vi "Process.vi"(8 "error in":errorcluster, 11 "MeasurementSMO":refnum<class "AFM_Litho_Plugin.IV.lvclass">) -> (0 "error out":errorcluster, 3 "MeasurementSMO out":refnum<class "AFM_Litho_Plugin.IV.lvclass">)   [LabVIEW 2019, in "AFM_Litho_Plugin.IV.lvclass"]
doc: "---------------------------------------------------------------\nJKI State Machine Objects™\nhttp://jki.net/state-machine-objects/\nCopyright (C) 2005-2015, JKI <info@jki.net>\nALL RIGHTS RESERVED"
uses:
  AFM_Litho_Plugin.IV.lvclass
  C:/Program Files (x86)/National Instruments/LabVIEW 2019/vi.lib/JKI/JKI SMO/SMO/SMO.lvclass
  C:/Program Files (x86)/National Instruments/LabVIEW 2019/vi.lib/JKI/JKI SMO/SMO.UI/SMO.UI.lvclass
  <vilib>/JKI/JKI SMO/SMO/Typedefs/Parent Call--Enum.ctl
  AFM_Litho_Plugin.IV.lvclass/AFM_Litho_Plugin.IV.ctl
  Typedefs/PrivateEvents--AFM_Litho_Plugin.IV.IV Run--Local.ctl
  <userlib>/LevyLab/Instrument Framework/SMOs/RemoteControl/RemoteControl.lvclass
  <userlib>/LevyLab/Instrument Framework/SMOs/RemoteControl/Typedefs/Message--Cluster.ctl
  <userlib>/LevyLab/Instrument Framework/SMOs/RemoteControl/Typedefs/PrivateEvents--RemoteControl.SendMessageToProcess.ctl
  Program Files (x86)/National Instruments/LabVIEW 2020/user.lib/LevyLab/Lockin-Multichannel/Instrument.DAQ/Typedefs/Get State-enum.ctl
  <vilib>/JKI/JKI SMO/SMO/SMO.lvclass/SMO.ctl
  <userlib>/LevyLab/Instrument Framework/SMOs/RemoteControl/Typedefs/RC Com Type--enum.ctl
  fb8dc625-7147-424d-9f65-00a13242d459.vi
  <vilib>/JKI/JKI SMO/SMO/Private/ReftoDVR--SMO.vi
  fb8dc625-7147-424d-9f65-00a13242d459.vi/a9304a9f-69c7-45ea-b89b-09982a2100b8.vi
  <vilib>/Utility/LVClass/Get LV Class Name.vi
  <vilib>/JDP Science/JSONtext/JSON text to Variant.vi
  <vilib>/JDP Science/JSONtext/LVClass Serializer/JSONtext LVClass Serializer.lvclass
  <vilib>/JKI/JKI SMO/SMO.UI/SMO.UI.lvclass
  <vilib>/JKI/JKI SMO/SMO/SMO.lvclass
  <userlib>/LevyLab/Lockin-Multichannel/Instrument.DAQ/Instrument.DAQ.lvclass
panel:
  out "Lock-in Connection":bool
  out "Incoming Command":string
  out "Start":dbl caption="Numeric"
  out "End":dbl caption="Numeric"
  out "Rate":dbl caption="Numeric"
  out "Cycles":u32 caption="Numeric"
  out "Pattern":T1(ring) caption="Enum"
  in  "Output Channel":u16(ring) caption="Ring" items=["Ring", "Item 1", "Item 2", "Item 3"]
  out "IV Plug-in Address":u32 caption="Numeric"
  in  "Lock-in Amplifier Address":string
  # "IV Curve Measurement Plugin"
  # "ipconfig /all"
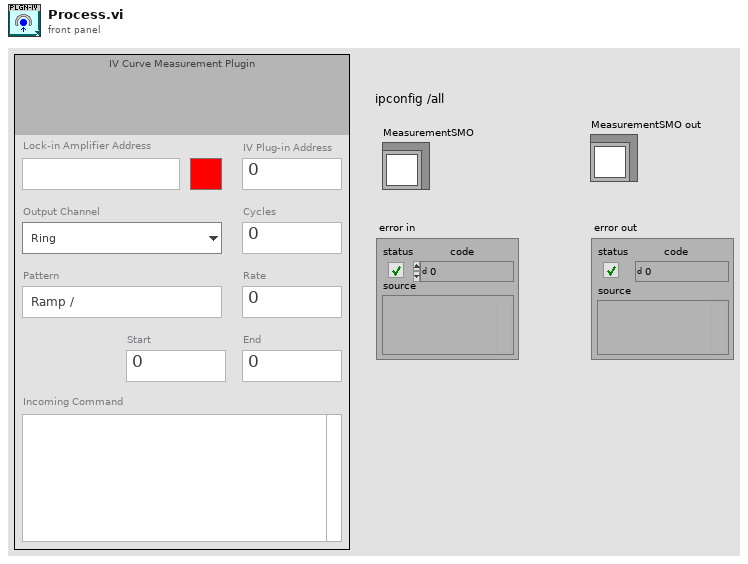
[diagram p1: front panel]
types:
  T1 = enum16{"Ramp /", "Ramp /\\", "Smooth Ramp _/", "Smooth Ramp _/\\_", "Frequency"}
  T2 = typedef "SMO.lvclass/Parent Call--Enum.ctl" = enum16{"Allows parent to run", "Does not request parent to run"}
  T3 = typedef "AFM_Litho_Plugin.IV.lvclass/PrivateEvents--AFM_Litho_Plugin.IV.IV Run--Local.ctl" = cluster{"Pattern":enum16{"Ramp /", "Ramp /\\", "Smooth Ramp _/", "Smooth Ramp _/\\_", "Frequency"}, "Cycles":dbl, "Rate":dbl, "End":dbl, "Start":dbl}
  T4 = enum32{"invalid app kind", "Development System", "Run Time System", "Student Edition", "Embedded LabVIEW", "Evaluation", "Custom"}
  T5 = typedef "Instrument.DAQ.lvclass/Get State-enum.ctl" = enum16{"idle", "created", "started", "stopped", "sweeping"}
  T6 = enum32{"Invalid", "Standard", "Closed", "Hidden", "Minimized", "Maximized"}
  T7 = enum32{"Bad", "Idle", "Run top level", "Running"}
  T8 = typedef "RemoteControl.lvclass/Message--Cluster.ctl" = cluster{"Command":string, "Data":variant, "ID":string}
  T9 = typedef "RemoteControl.lvclass/RC Com Type--enum.ctl" = enum16{"RC", "STM", "ZMQ"}
  T10 = cluster{"Shift":bool, "Ctrl":bool, "Alt":bool, "Cmd":bool, "Opt":bool}
  T11 = typedef "RemoteControl.lvclass/PrivateEvents--RemoteControl.SendMessageToProcess.ctl" = cluster{"Message":T8}
  T12 = cluster{"Core":cluster{"Current VI Reference":refnum<vi>, "Close Panel on Exit?":bool, "error":errorcluster}, "Self Reference":refnum<class "AFM_Litho_Plugin.IV.lvclass">, "Voltage Channel":u16, "Lockin Address":string, "Plugin Address":i32, "Server":refnum<class "RemoteControl.lvclass">, "Server Req":T8, "Server Rep":T11, "Cycles":dbl, "Status":T5, "IV Run":T3, "IV Status":string, "Command History":string, "Command Message":string, "Start Status":string}
  T13 = cluster{"Current VI Reference":refnum<vi>, "Close Panel on Exit?":bool, "error":errorcluster}
  T14 = typedef "RemoteControl.lvclass/PublicEvents--Cluster.ctl" = cluster{"SendMessageFromProcess":refnum<user-event>}
  T15 = typedef "AFM_Litho_Plugin.IV.lvclass/PrivateEvents--Cluster.ctl" = cluster{"IV Run--Local":refnum<user-event>, "IV Status--Local":refnum<user-event>}
  T16 = typedef "SMO.lvclass/Protected Events.ctl" = cluster{"StopProcesses":refnum<user-event>, "AbortProcesses":refnum<user-event>, "Config Changed":refnum<user-event>, "Dependency":refnum<user-event>}
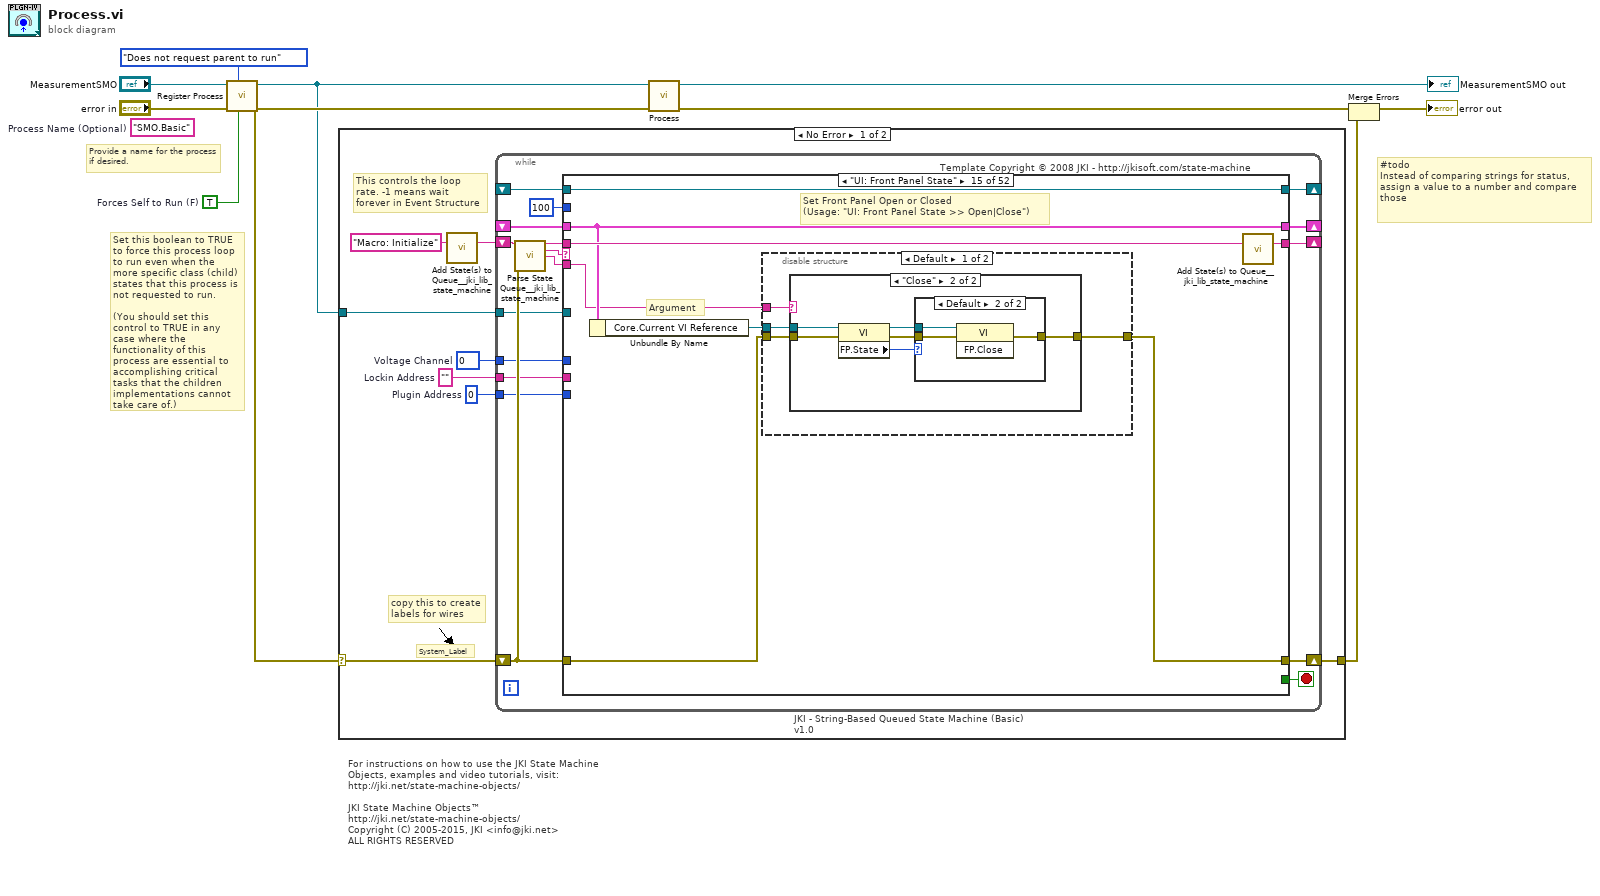
[diagram p0: block diagram]
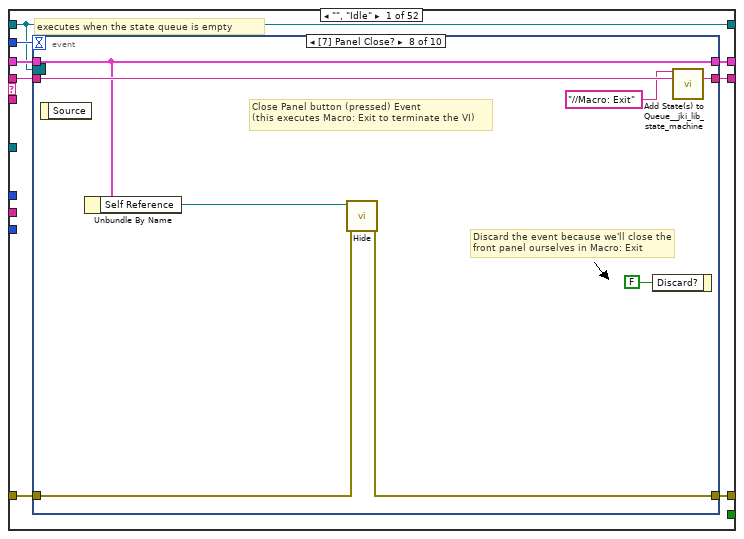
[diagram p2: hidden frame]
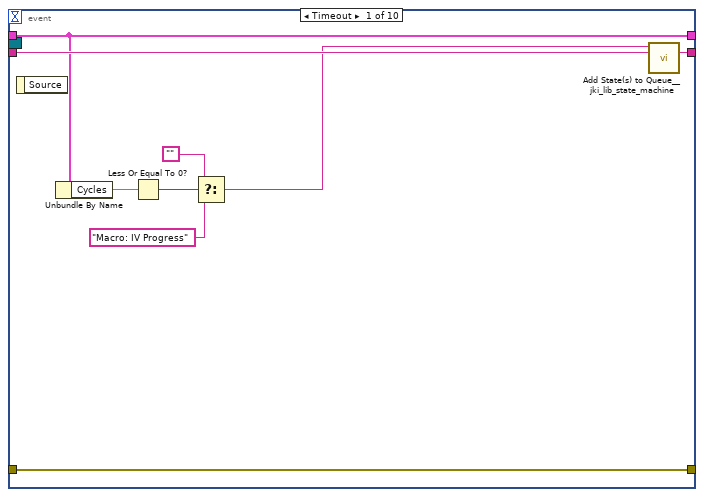
[diagram p3: hidden frame]
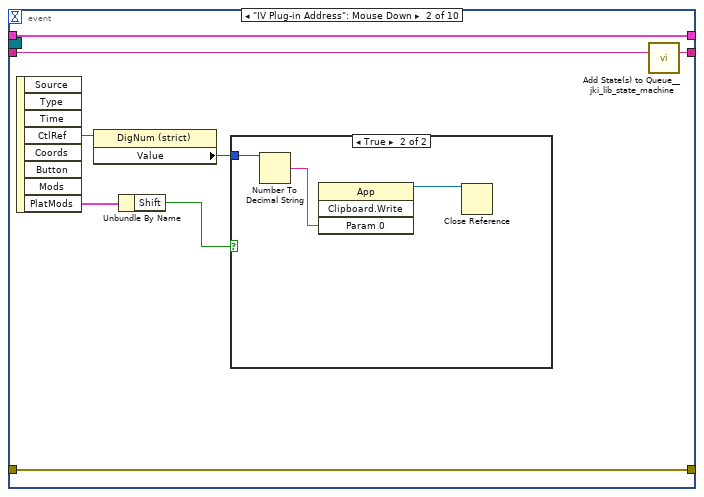
[diagram p4: hidden frame]
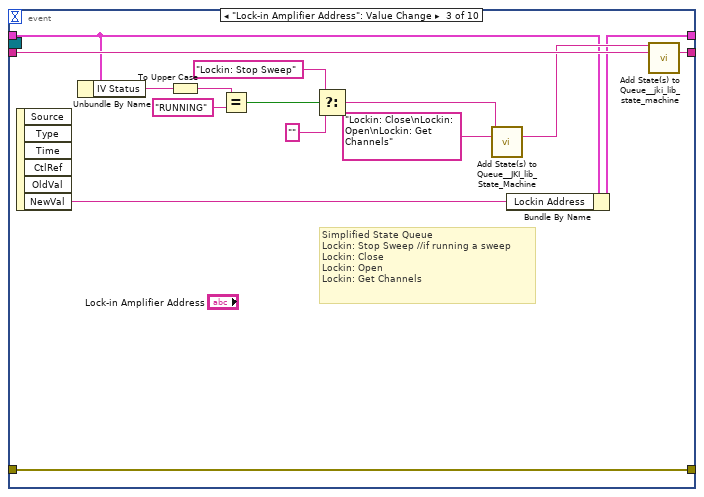
[diagram p6: hidden frame]
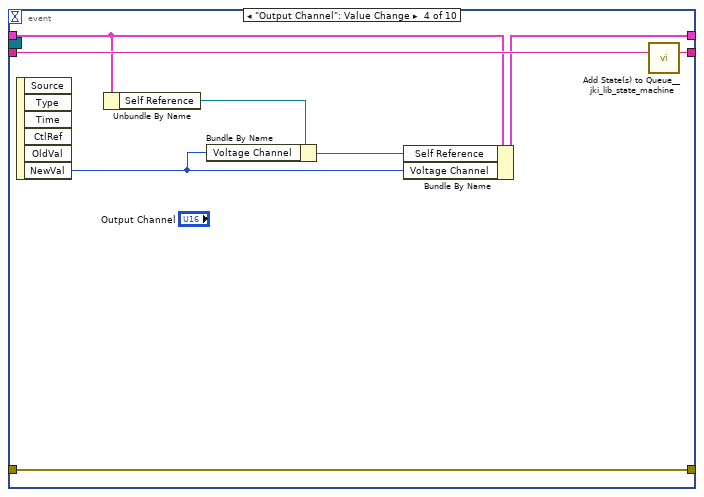
[diagram p7: hidden frame]
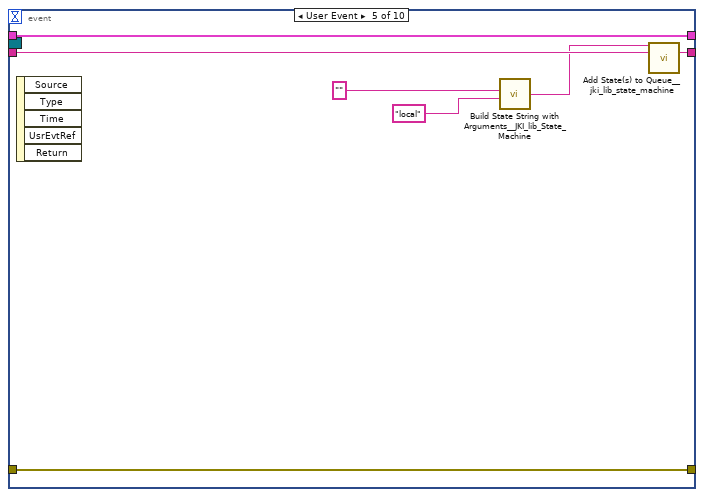
[diagram p8: hidden frame]
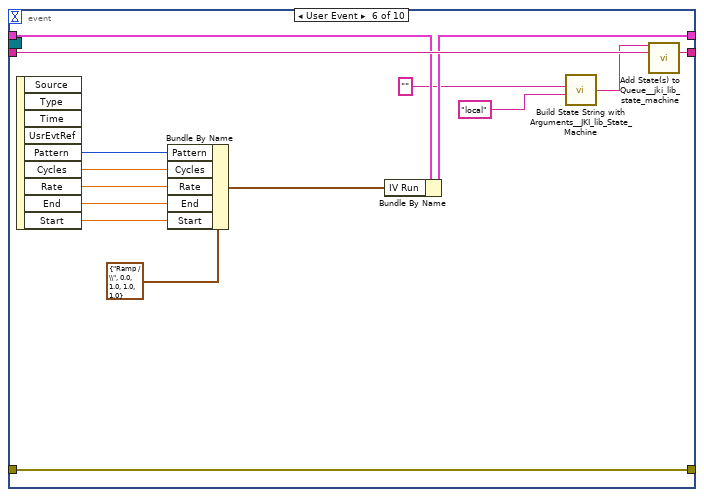
[diagram p9: hidden frame]
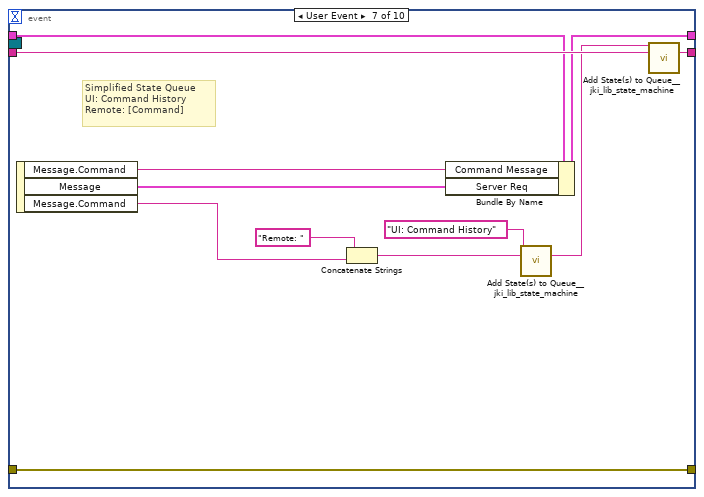
[diagram p10: hidden frame]
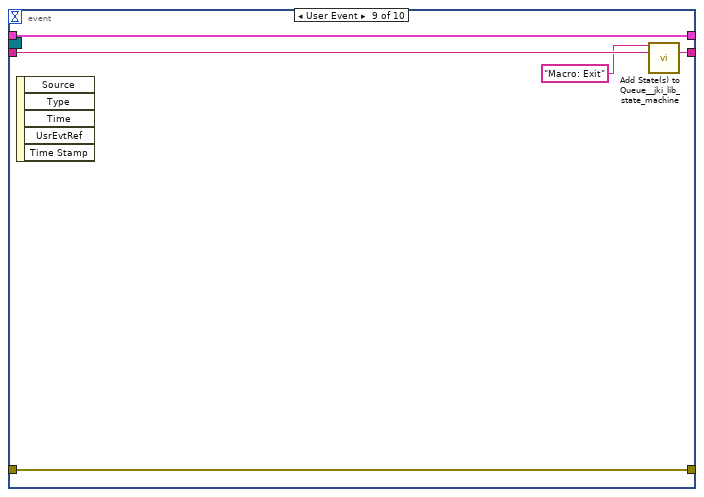
[diagram p11: hidden frame]
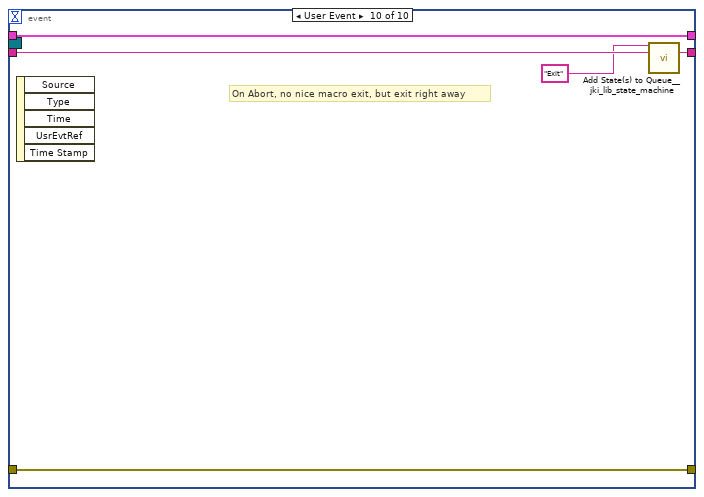
[diagram p12: hidden frame]
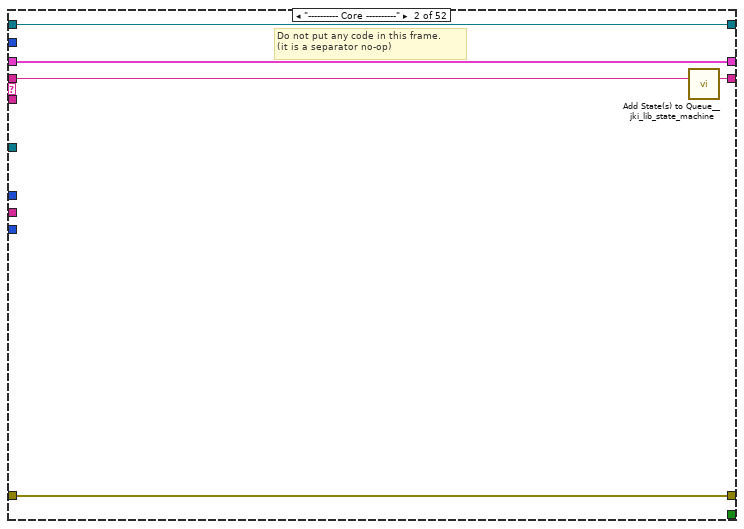
[diagram p13: hidden frame]
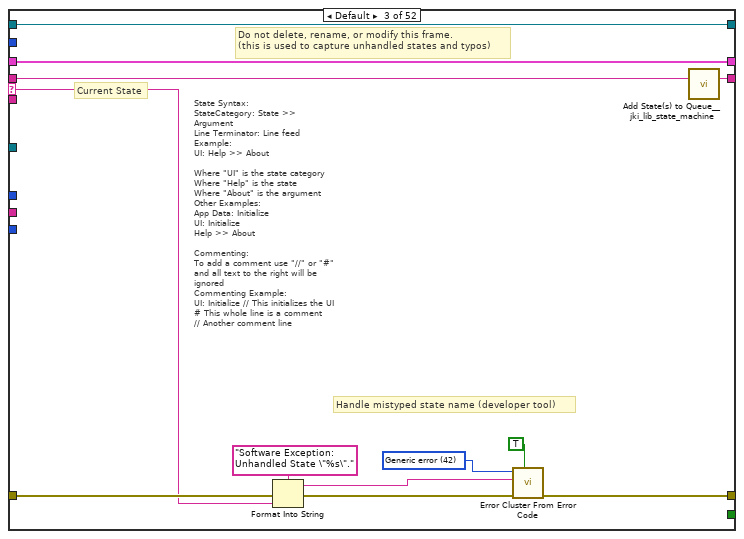
[diagram p14: hidden frame]
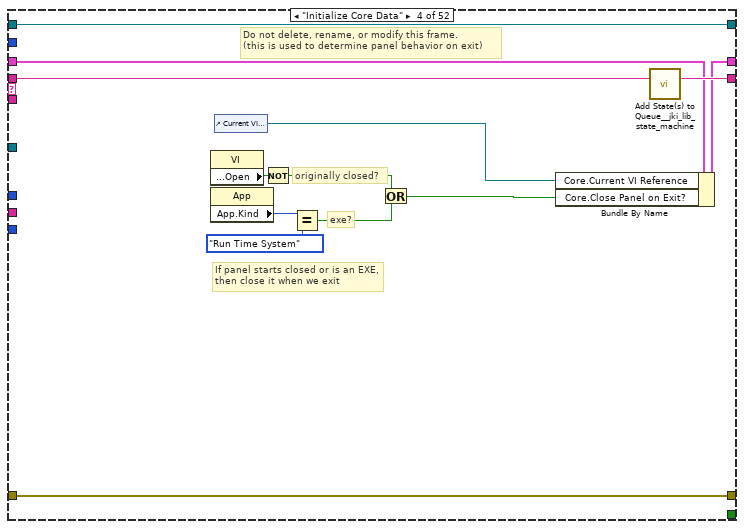
[diagram p15: hidden frame]
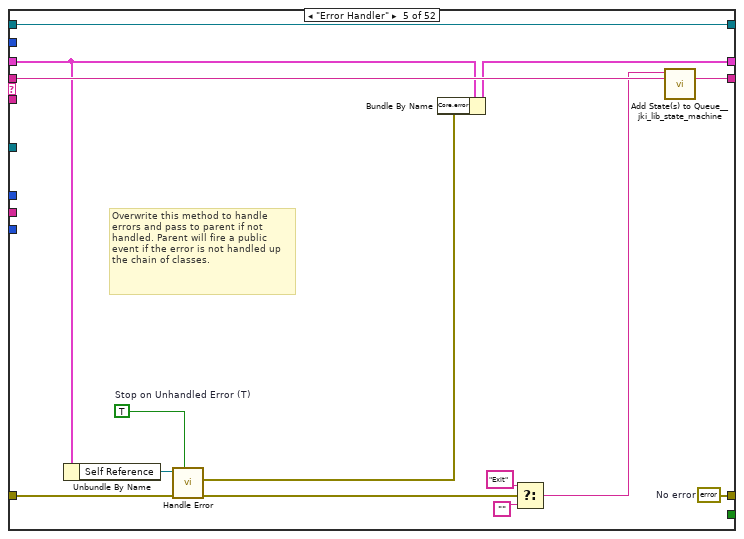
[diagram p16: hidden frame]
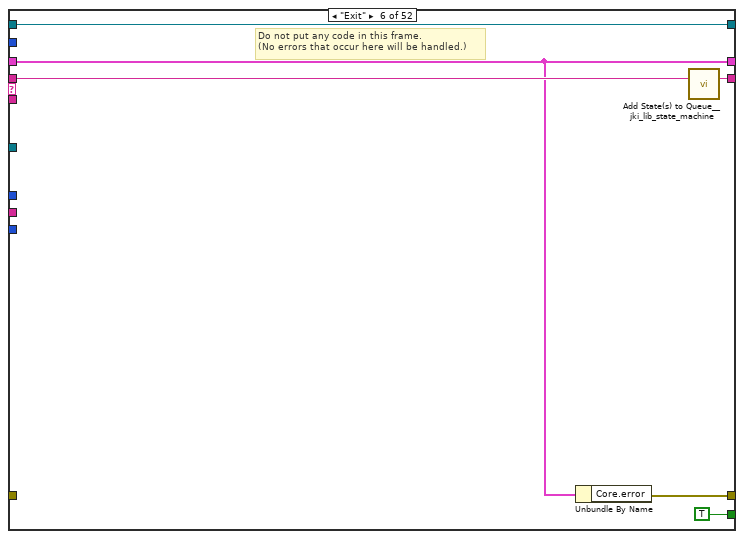
[diagram p17: hidden frame]
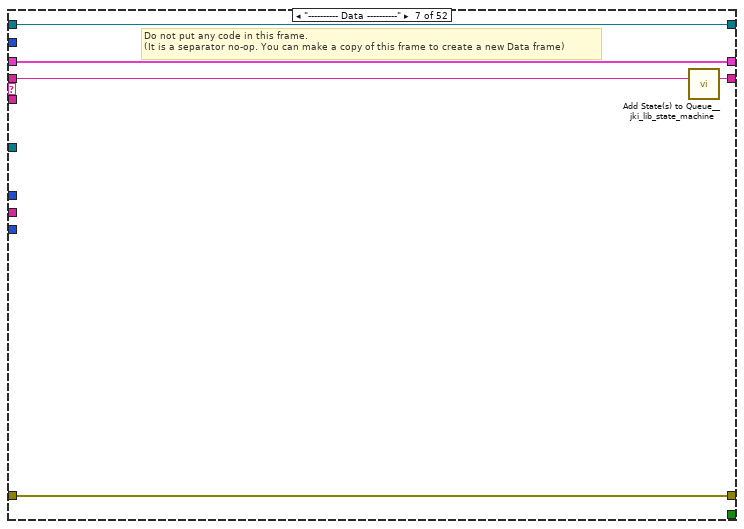
[diagram p18: hidden frame]
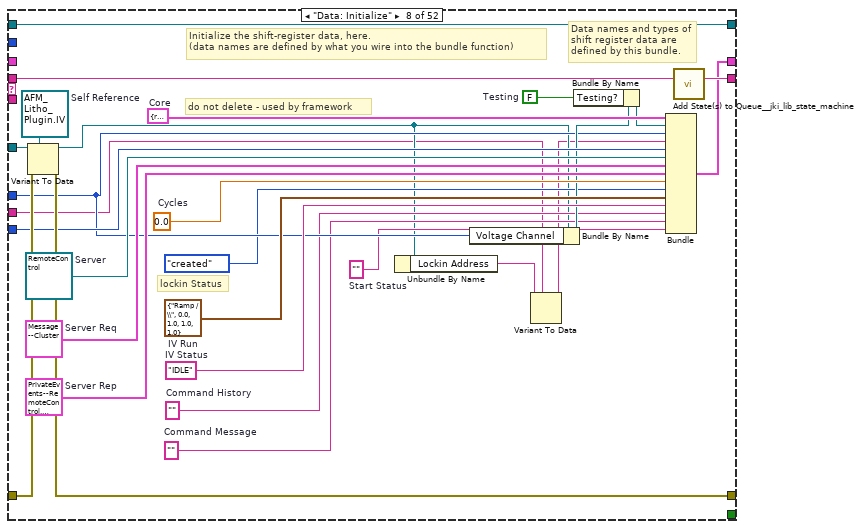
[diagram p19: hidden frame]
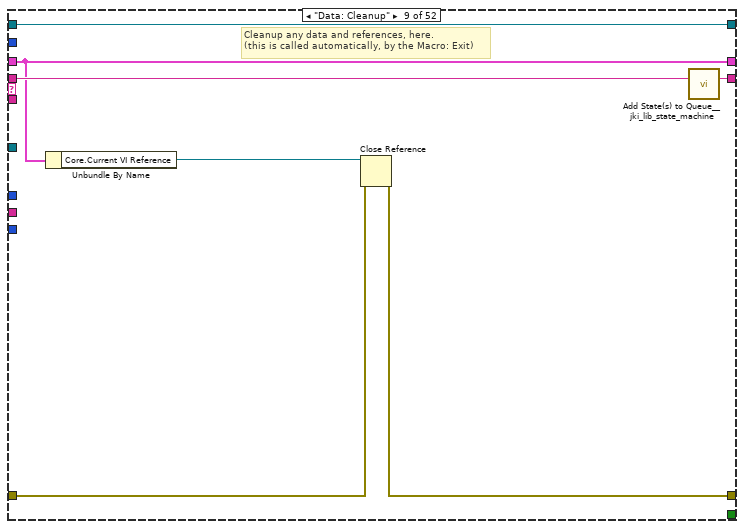
[diagram p20: hidden frame]
diagram:
  w1 = TRUE  # Forces Self to Run (F)
  (unwired) "SMO.Basic"  # Process Name (Optional)
  # "#todo\nInstead of comparing strings for status, assign a value to a number and compare those"
  # "Provide a name for the process\nif desired."
  # "Set this boolean to TRUE to force this process loop to run even when the more specific class (child) states that this process is not requested to run.\n\n(You should set this control to TRUE in any case where the functionality of this process are essential to accomplishing critical tasks that the children implementations cannot take care of.)"
  # "For instructions on how to use the JKI State Machine Objects, examples and video tutorials, visit:\nhttp://jki.net/state-machine-objects/\n\nJKI State Machine Objects™\nhttp://jki.net/state-machine-objects/\nCopyright (C) 2005-2015, JKI <info@jki.net>\nALL RIGHTS RESERVED"
  n1 = call <vilib>:"Register Process.vi"("Forces Self to Run (F)"=w1, "Parent Call"=Parent_Call--Enum."Does not request parent to run", "error in (no error)"="error in", "SMO"="MeasurementSMO") -> ("error out"=w7:errorcluster, "SMO out"=w6:refnum<class "AFM_Litho_Plugin.IV.lvclass">)  [unwired: 6 in]
  n2 = case shown="No Error" w7 {
    selector: w7 -> [w15 w773]
    tunnel: w6 -> [w16 _]
    tunnel: [w14 w773] -> w3
    frame No Error {
      w11 = 0  # Plugin Address
      w12 = ""  # Lockin Address
      w13 = u16 0 items=[""]  # Voltage Channel
      # "copy this to create labels for wires"
      # "This controls the loop rate. -1 means wait forever in Event Structure"
      # "System_Label"
      n3 = call <vilib>:"Add State(s) to Queue__jki_lib_state_machine.vi"("State(s) in (\"\")"="Macro: Initialize") -> ("States Out"=w18:string)  [unwired: 14 in]
      n4 = while "JKI - String-Based Queued State Machine (Basic) v1.0" {
        shift-right: [w28] -> _
        shift-left: _ -> [w27]
        shift-right: [w31] -> w14
        shift-left: w15 -> [w25]
        shift-right: [w30] -> _
        shift-left: w18 -> [w32]
        tunnel: w16 -> [w24]
        shift-right: [w23] -> _
        shift-left: _ -> [w22]
        tunnel: w13 -> [w21]
        tunnel: w12 -> [w20]
        tunnel: w11 -> [w19]
        stop <- w29 stop-if-true
        # "Template Copyright © 2008 JKI - http://jkisoft.com/state-machine"
        n5 = call <vilib>:"Parse State Queue__jki_lib_state_machine.vi"("State Queue"=w32, "Error In (no error)"=w25) -> ("Remaining States"=w34:string, "Current State"=w35:string, "Arguments"=w33:string)  [unwired: 11 in]
        n6 = case shown="\"UI: Front Panel State\"" w35 {
          selector: w35 -> [_ _ w145 _ _ _ _ _ _ _ _ _ _ _ _ _ _ _ _ _ _ _ _ _ _ _ _ _ _ _ _ _ _ _ _ _ _ _ _ _ _ _ _ _ _ _ _ _ _ _ _ _]
          tunnel: w34 -> [w43 w143 w149 w168 w182 w188 w193 w221 w228 w233 w245 w272 w296 w303 w319 w351 w357 w363 w377 w391 w396 w407 w412 w427 w433 w440 w442 w467 w479 w497 w507 w516 w526 w537 w547 w556 w563 w574 w595 w604 w613 w622 w632 w642 w664 w674 w693 w718 w729 w734 w752 w772]
          tunnel: w33 -> [_ _ _ _ _ _ _ _ _ _ w238 _ _ w297 w313 _ _ _ _ _ _ _ _ _ _ _ _ _ _ w492 _ _ _ _ _ _ _ _ _ _ _ _ _ w638 _ _ _ _ _ _ _ _]
          tunnel: w27 -> [w41 w140 w147 w159 w176 w184 w190 _ w223 w230 w235 w262 w291 w301 w315 w348 w354 w360 w373 w382 w393 w404 w409 w419 w431 w435 w451 w463 w475 w487 w498 w512 w522 w532 w543 w552 w558 w570 w592 w597 w609 w618 w623 w636 w655 w666 w685 w695 w723 w732 w746 w765]
          tunnel: [w40 w141 w151 w165 w177 w183 w191 w217 w224 w231 w241 w264 w285 w298 w316 w349 w355 w361 w375 w389 w394 w398 w410 w422 w429 w437 w448 w455 w468 w494 w499 w508 w518 w529 w541 w550 w560 w566 w578 w600 w606 w615 w629 w639 w661 w671 w690 w703 w726 w730 w749 w769] -> w31
          tunnel: w25 -> [w39 w141 w150 w165 w178 _ w191 w218 w225 w231 w240 w248 w292 w299 w317 w349 w355 w361 w375 w389 w394 w399 w410 w423 w429 w437 w449 w461 w472 w493 w500 w509 w519 w528 w542 w551 w560 w565 w577 w599 w605 w614 w629 w639 w661 w671 w690 w709 w726 w730 w749 w769]
          tunnel: [w42 w142 w148 w167 w181 w187 w192 w220 w227 w232 w244 w271 w295 w302 w318 w350 w356 w362 w376 w390 w395 w406 w411 w426 w432 w439 w454 w466 w478 w496 w506 w515 w525 w536 w546 w555 w562 w573 w594 w603 w612 w621 w631 w641 w663 w673 w692 w717 w728 w733 w751 w771] -> w30
          tunnel: [_ _ _ _ _ TRUE _ _ _ _ _ _ _ _ _ _ _ _ _ _ _ _ _ _ _ _ _ _ _ _ _ _ _ _ _ _ _ _ _ _ _ _ _ _ _ _ _ _ _ _ _ _] -> w29
          tunnel: [w38 w140 w147 w166 w175 w184 w190 w219 w223 w230 w236 w263 w291 w301 w315 w348 w354 w360 w373 w382 w393 w404 w409 w419 w431 w436 w452 w464 w476 w488 w504 w513 w523 w533 w544 w553 w559 w571 w591 w598 w610 w619 w623 w637 w655 w666 w686 w710 w723 w732 w747 w765] -> w28
          tunnel: 100 ("Timeout") -> [w37 _ _ _ _ _ _ _ _ _ _ _ _ _ _ _ _ _ _ _ _ _ _ _ _ _ _ _ _ _ _ _ _ _ _ _ _ _ _ _ _ _ _ _ _ _ _ _ _ _ _ _]
          tunnel: w24 -> [_ _ _ _ _ _ _ w215 _ _ _ _ _ _ _ _ _ _ _ _ _ _ _ _ _ _ _ _ _ _ _ _ _ _ _ _ _ _ _ _ _ _ _ _ _ _ _ _ _ _ _ _]
          tunnel: [w36 w139 w144 w156 w180 w185 w189 w214 w222 w229 w243 w270 w294 w300 w312 w347 w353 w359 w374 w383 w392 w405 w408 w425 w430 w438 w453 w465 w477 w495 w505 w514 w524 w535 w545 w554 w561 w572 w593 w602 w611 w620 w630 w640 w662 w672 w691 w716 w727 w731 w750 w770] -> w23
          tunnel: w22 -> [w36 w139 w144 w156 w180 w185 w189 w214 w222 w229 w243 w270 w294 w300 w312 w347 w353 w359 w374 w383 w392 w405 w408 _ w430 w438 w453 w465 w477 w495 w505 w514 w524 w535 w545 w554 w561 w572 w593 w602 w611 w620 w630 w640 w662 w672 w691 w716 w727 w731 w750 w770]
          tunnel: w21 -> [_ _ _ _ _ _ _ w202 _ _ _ _ _ _ _ _ _ _ _ _ _ _ _ _ _ _ _ _ _ _ _ _ _ _ _ _ _ _ _ _ _ _ _ _ _ _ _ _ _ _ _ _]
          tunnel: w20 -> [_ _ _ _ _ _ _ w195 _ _ _ _ _ _ _ _ _ _ _ _ _ _ _ _ _ _ _ _ _ _ _ _ _ _ _ _ _ _ _ _ _ _ _ _ _ _ _ _ _ _ _ _]
          tunnel: w19 -> [_ _ _ _ _ _ _ w212 _ _ _ _ _ _ _ _ _ _ _ _ _ _ _ _ _ _ _ _ _ _ _ _ _ _ _ _ _ _ _ _ _ _ _ _ _ _ _ _ _ _ _ _]
          frame "", "Idle" {
            # "executes when the state queue is empty"
            n7 = event shown="[7] Panel Close?" {
              selector: w36 -> [_ _ _ _ _ _ _ _ _ _]
              dyn-events: _ -> [_ _ _ _ _ _ _ _ _ _]
              timeout: w37 -> [_ _ _ _ _ _ _ _ _ _]
              tunnel: w43 -> [w52 w60 w78 w86 w93 w108 w120 w128 w133 w138]
              tunnel: [w51 w59 w77 w85 w92 w107 w119 w127 w132 w137] -> w42
              tunnel: w41 -> [w49 w57 w67 w82 w91 w98 w115 w124 w130 w135]
              tunnel: [w50 w58 w76 w84 w90 w106 w114 w122 w131 w136] -> w40
              tunnel: w39 -> [w50 w58 w76 w84 w90 w106 w114 w123 w131 w136]
              tunnel: [w49 w57 w68 w83 w91 w99 w118 w124 w130 w135] -> w38
              event Timeout {
                n8 = event-data() -> ()  [unwired: 1 in, 1 out]
                n9 = Unbundle By Name(w49) -> ("Cycles"=w48:dbl)
                n10 = Less Or Equal To 0?(x=w48) -> (x <= 0?=w47:bool)
                n11 = Select(t="", s=w47, f="Macro: IV Progress") -> (s? t:f=w44:string)
                n12 = call <vilib>:"Add State(s) to Queue__jki_lib_state_machine.vi"("State(s) in Front (\"\")"=w44, "State(s) in (\"\")"=w52) -> ("States Out"=w51:string)  [unwired: 13 in]
              }
              event "IV Plug-in Address": Mouse Down {
                n13 = event-data() -> ("CtlRef"=w55:refnum<vi>, "PlatMods"=w56:T10)  [unwired: 1 in, 6 out]
                n14 = property class="DigNum (strict)"(reference=w55) -> ("Value"=w54:u32)  [unwired: 1 in, 2 out]
                n15 = Unbundle By Name(w56) -> ("Shift"=w53:bool)
                n16 = case shown="True" w53 {
                  tunnel: w54 -> [_ w63]
                  frame False {
                  }
                  frame True {
                    n17 = Number To Decimal String(number=w63) -> (decimal integer string=w62:string)  [unwired: 1 in]
                    n18 = invoke class="App" method="Clipboard.Write"("Param 0"=w62) -> (reference out=w61:refnum<vi>)  [unwired: 3 in, 3 out]
                    n19 = Close Reference(reference=w61) -> ()  [unwired: 1 in, 1 out]
                  }
                }
                n20 = call <vilib>:"Add State(s) to Queue__jki_lib_state_machine.vi"("State(s) in (\"\")"=w60) -> ("States Out"=w59:string)  [unwired: 14 in]
              }
              event "Lock-in Amplifier Address": Value Change {
                # "Simplified State Queue\nLockin: Stop Sweep //if running a sweep\nLockin: Close\nLockin: Open\nLockin: Get Channels"
                n21 = event-data() -> ("NewVal"=w66:string)  [unwired: 1 in, 5 out]
                n22 = Unbundle By Name(w67) -> ("IV Status"=w75:string)
                n23 = To Upper Case(1:w75) -> (0:w64:string)
                n24 = Equal?(x=w64, y="RUNNING") -> (x = y?=w73:bool)
                n25 = Select(t="Lockin: Stop Sweep", s=w73, f="") -> (s? t:f=w71:string)
                n26 = call <vilib>:"Add State(s) to Queue__JKI_lib_State_Machine.vi"("State(s) in Front (\"\")"=w71, "State(s) in (\"\")"="Lockin: Close\nLockin: Open\nLockin: Get Channels" ("State(s) in (\"\")")) -> ("States Out"=w69:string)  [unwired: 13 in]
                n27 = Bundle By Name(cluster=w67, "Lockin Address"=w66) -> (w68:T12)
                n28 = call <vilib>:"Add State(s) to Queue__jki_lib_state_machine.vi"("State(s) in Front (\"\")"=w69, "State(s) in (\"\")"=w78) -> ("States Out"=w77:string)  [unwired: 13 in]
              }
              event "Output Channel": Value Change {
                n29 = event-data() -> ("NewVal"=w80:u16)  [unwired: 1 in, 5 out]
                n30 = Unbundle By Name(w82) -> ("Self Reference"=w81:refnum<class "AFM_Litho_Plugin.IV.lvclass">)
                n31 = Bundle By Name(cluster=w81, "Voltage Channel"=w80) -> (w79:refnum<class "AFM_Litho_Plugin.IV.lvclass">)
                n32 = Bundle By Name(cluster=w82, "Self Reference"=w79, "Voltage Channel"=w80) -> (w83:T12)
                n33 = call <vilib>:"Add State(s) to Queue__jki_lib_state_machine.vi"("State(s) in (\"\")"=w86) -> ("States Out"=w85:string)  [unwired: 14 in]
              }
              event User Event {
                n34 = event-data() -> ()  [unwired: 1 in, 5 out]
                n35 = call <vilib>:"Build State String with Arguments__JKI_lib_State_Machine.vi"("Arguments (\"\")"="local" ("Arguments (\"\")"), "State"="") -> ("State with Arguments"=w87:string)  [unwired: 4 in]
                n36 = call <vilib>:"Add State(s) to Queue__jki_lib_state_machine.vi"("State(s) in Front (\"\")"=w87, "State(s) in (\"\")"=w93) -> ("States Out"=w92:string)  [unwired: 13 in]
              }
              event User Event {
                n37 = event-data() -> ("Pattern"=w100:T1, "Cycles"=w101:dbl, "Rate"=w102:dbl, "End"=w103:dbl, "Start"=w104:dbl)  [unwired: 1 in, 4 out]
                n38 = Bundle By Name(cluster=T3 {"Pattern"=enum."Ramp /\\", "Cycles"=0.0, "Rate"=1.0, "End"=1.0, "Start"=1.0} ("IV Run--Local"), "Pattern"=w100, "Cycles"=w101, "Rate"=w102, "End"=w103, "Start"=w104) -> (w97:T3)
                n39 = Bundle By Name(cluster=w98, "IV Run"=w97) -> (w99:T12)
                n40 = call <vilib>:"Build State String with Arguments__JKI_lib_State_Machine.vi"("Arguments (\"\")"="local" ("Arguments (\"\")"), "State"="") -> ("State with Arguments"=w94:string)  [unwired: 4 in]
                n41 = call <vilib>:"Add State(s) to Queue__jki_lib_state_machine.vi"("State(s) in Front (\"\")"=w94, "State(s) in (\"\")"=w108) -> ("States Out"=w107:string)  [unwired: 13 in]
              }
              event User Event {
                # "Simplified State Queue\nUI: Command History\nRemote: [Command]"
                n42 = event-data() -> ("Message.Command"=w109:string, "Message"=w117:T8, "Message.Command"=w116:string)  [unwired: 1 in]
                n43 = Concatenate Strings("Remote: ", w116) -> (w113:string)
                n44 = Bundle By Name(cluster=w115, "Command Message"=w109, "Server Req"=w117) -> (w118:T12)
                n45 = call <vilib>:"Add State(s) to Queue__jki_lib_state_machine.vi"("State(s) in Front (\"\")"="UI: Command History", "State(s) in (\"\")"=w113) -> ("States Out"=w111:string)  [unwired: 13 in]
                n46 = call <vilib>:"Add State(s) to Queue__jki_lib_state_machine.vi"("State(s) in Front (\"\")"=w111, "State(s) in (\"\")"=w120) -> ("States Out"=w119:string)  [unwired: 13 in]
              }
              event Panel Close? {
                # "Discard the event because we'll close the front panel ourselves in Macro: Exit"
                # "Close Panel button (pressed) Event\n(this executes Macro: Exit to terminate the VI)"
                n47 = event-data() -> ()  [unwired: 1 in, 1 out]
                n48 = Unbundle By Name(w124) -> ("Self Reference"=w121:refnum<class "AFM_Litho_Plugin.IV.lvclass">)
                n49 = call <vilib>:"Hide.vi"("error in (no error)"=w123, "SMO.UI"=w121) -> ("error out"=w122:errorcluster)  [unwired: 8 in, 1 out]
                n50 = event-data("Discard?"=FALSE) -> ()  [unwired: 1 in, 1 out]
                n51 = call <vilib>:"Add State(s) to Queue__jki_lib_state_machine.vi"("State(s) in Front (\"\")"="//Macro: Exit", "State(s) in (\"\")"=w128) -> ("States Out"=w127:string)  [unwired: 13 in]
              }
              event User Event {
                n52 = event-data() -> ()  [unwired: 1 in, 5 out]
                n53 = call <vilib>:"Add State(s) to Queue__jki_lib_state_machine.vi"("State(s) in Front (\"\")"="Macro: Exit", "State(s) in (\"\")"=w133) -> ("States Out"=w132:string)  [unwired: 13 in]
              }
              event User Event {
                # "On Abort, no nice macro exit, but exit right away"
                n54 = event-data() -> ()  [unwired: 1 in, 5 out]
                n55 = call <vilib>:"Add State(s) to Queue__jki_lib_state_machine.vi"("State(s) in Front (\"\")"="Exit", "State(s) in (\"\")"=w138) -> ("States Out"=w137:string)  [unwired: 13 in]
              }
            }
          }
          frame "---------- Core ----------" {
            # "Do not put any code in this frame.\n(it is a separator no-op)"
            n56 = call <vilib>:"Add State(s) to Queue__jki_lib_state_machine.vi"("State(s) in (\"\")"=w143) -> ("States Out"=w142:string)  [unwired: 14 in]
          }
          frame Default {
            w154 = 42 items=["No error", "Argument error", "Memory is full", "Out of zone", "End of file", "File already open", "Generic file I/O error", "File not found", "File permission error", "Disk is full", "Duplicate path", "Too many files open", "System feature not enabled", "Resource file not found", "Cannot add resource", "Resource not found", "Image not found", "Image memory error", "Pen does not exist", "Config type invalid", "Config token not found", "Config parse error", "Config memory error", "Bad external code format", "Bad external code offset", "External code not present", "Null window", "Destroy window error", "Null menu", "Print aborted", "Bad print record", "Print driver error", "Windows error during printing", "Memory error during printing", "Print dialog error", "Generic print error", "Invalid device refnum", "Device not found", "Device parameter error", "Device unit error", "Cannot open device", "Device call aborted", "Generic error", "Cancelled by user", "Object ID too low", "Object ID too high", "Object not in heap", "Unknown heap", "Unknown object (invalid DefProc)", "Unknown object (DefProc not in table)", "Message out of range", "Invalid (null) method", "Unknown message", "Manager call not supported", "Bad address", "Network operation in progress", "Network operation timed out", "Connection is busy", "Network attribute not supported", "Network error", "Address in use", "System out of memory", "Connection aborted", "Connection refused", "Not connected", "Already connected", "Connection closed", "Initialization error (interapplication manager)", "Bad occurrence", "Wait on unbound occurrence handler", "Occurrence queue overflow", "Datalog type conflict", "Unused", "Unrecognized type (interapplication manager)", "Memory corrupt", "Failed to make temporary DLL", "Old CIN version", "Drag socket not found", "Failed to load drop-object", "Failed to register OLE object", "Failed to release OLE object", "Format specifier type mismatch", "Unknown format specifier", "Too few format specifiers", "Too many format specifiers", "Scan failed", "Newer CIN version", "Error converting to variant", "Runtime menu error", "Password tampered", "Variant attribute not found", "Incompatible variant data type", "Event data is not available", "Event Store is not present", "Occurrence is not found", "Event Queue is not created", "Event info is not available", "Refnum passed is NULL", "Error retrieving Class GUID", "Error retrieving CoClass GUID", "Error retrieving TypeLib GUID.", "Bad built application magic bytes.", "Specific driver is different from the specific driver associated with the Logical Name.", "There is no session opened to the class driver.", "Max Error", "MAX - Error with config objects", "MAX - Error loading configuration", "MAX - Group not supported"]
            # "State Syntax:\nStateCategory: State >> Argument\nLine Terminator: Line feed\nExample:\nUI: Help >> About\n\nWhere \"UI\" is the state category\nWhere \"Help\" is the state\nWhere \"About\" is the argument\nOther Examples:\nApp Data: Initialize\nUI: Initialize\nHelp >> About\n\nCommenting:\nTo add a comment use \"//\" or \"#\" and all text to the right will be ignored\nCommenting Example:\nUI: Initialize // This initializes the UI\n# This whole line is a comment\n// Another comment line"
            # "Current State"
            # "Do not delete, rename, or modify this frame.\n(this is used to capture unhandled states and typos)"
            # "Handle mistyped state name (developer tool)"
            n57 = Format Into String(format string="Software Exception: Unhandled State \"%s\"." ("message"), error in=w150, w145) -> (resulting string=w153:string, error out=w152:errorcluster)  [unwired: 1 in]
            n58 = call <vilib>:"Error Cluster From Error Code.vi"("show call chain? (False)"=TRUE, "error in (no error)"=w152, "error message (\"\")"=w153, "error code (0)"=w154) -> ("error out"=w151:errorcluster)  [unwired: 5 in]
            n59 = call <vilib>:"Add State(s) to Queue__jki_lib_state_machine.vi"("State(s) in (\"\")"=w149) -> ("States Out"=w148:string)  [unwired: 14 in]
          }
          frame "Initialize Core Data" {
            # "Do not delete, rename, or modify this frame.\n(this is used to determine panel behavior on exit)"
            # "originally closed?"
            # "exe?"
            # "If panel starts closed or is an EXE, then close it when we exit"
            n60 = property class="VI"() -> ("Front Panel.Open"=w164:bool)  [unwired: 2 in, 2 out]
            n61 = property class="App"() -> ("App.Kind"=w163:T4)  [unwired: 2 in, 2 out]
            n62 = control-ref of="Current VI Reference"() -> (w157:refnum<vi>)
            n63 = Not(x=w164) -> (.not. x?=w161:bool)
            n64 = Equal?(x=w163, y=T4."Run Time System" ("Application:Kind")) -> (x = y?=w160:bool)
            n65 = Or(x=w161, y=w160) -> (x .or. y?=w158:bool)
            n66 = Bundle By Name(cluster=w159, "Core.Current VI Reference"=w157, "Core.Close Panel on Exit?"=w158) -> (w166:T12)
            n67 = call <vilib>:"Add State(s) to Queue__jki_lib_state_machine.vi"("State(s) in (\"\")"=w168) -> ("States Out"=w167:string)  [unwired: 14 in]
          }
          frame "Error Handler" {
            w169 = TRUE  # Stop on Unhandled Error (T)
            w177 = errorcluster {"status"=FALSE, "code"=0, "source"=""}  # No error
            # "Overwrite this method to handle errors and pass to parent if not handled. Parent will fire a public event if the error is not handled up the chain of classes."
            n68 = Unbundle By Name(w176) -> ("Self Reference"=w179:refnum<class "AFM_Litho_Plugin.IV.lvclass">)
            n69 = call-dynamic "Handle Error.vi"("Stop on Unhandled Error (T)"=w169, "error in"=w178, "SMO"=w179) -> ("handling error"=w170:errorcluster, "Unhandled error"=w173:errorcluster)  [unwired: 6 in, 1 out]
            n70 = Bundle By Name(cluster=w176, "Core.error"=w173) -> (w175:T12)
            n71 = Select(t="Exit", s=w170, f="") -> (s? t:f=w174:string)
            n72 = call <vilib>:"Add State(s) to Queue__jki_lib_state_machine.vi"("State(s) in Front (\"\")"=w174, "State(s) in (\"\")"=w182) -> ("States Out"=w181:string)  [unwired: 13 in]
          }
          frame "Exit" {
            # "Do not put any code in this frame.\n(No errors that occur here will be handled.)"
            n73 = Unbundle By Name(w184) -> ("Core.error"=w183:errorcluster)
            n74 = call <vilib>:"Add State(s) to Queue__jki_lib_state_machine.vi"("State(s) in (\"\")"=w188) -> ("States Out"=w187:string)  [unwired: 14 in]
          }
          frame "---------- Data ----------" {
            # "Do not put any code in this frame.\n(It is a separator no-op. You can make a copy of this frame to create a new Data frame)"
            n75 = call <vilib>:"Add State(s) to Queue__jki_lib_state_machine.vi"("State(s) in (\"\")"=w193) -> ("States Out"=w192:string)  [unwired: 14 in]
          }
          frame "Data: Initialize" {
            w198 = ""  # Start Status
            w199 = ""  # Command Message
            w201 = ""  # Command History
            w204 = "IDLE"  # IV Status
            w205 = FALSE  # Testing
            w207 = T3 {"Pattern"=enum."Ramp /\\", "Cycles"=0.0, "Rate"=1.0, "End"=1.0, "Start"=1.0}  # IV Run
            w208 = 0.0  # Cycles
            w209 = T11 {"Message"={"Command"="", "Data"=variant(string ""), "ID"=""}}  # Server Rep
            w210 = T8 {"Command"="", "Data"=variant, "ID"=""}  # Server Req
            w211 = refnum<class "RemoteControl.lvclass"> refnum  # Server
            w213 = T13 {"Current VI Reference"=refnum, "Close Panel on Exit?"=FALSE, "error"={"status"=FALSE, "code"=0, "source"=""}}  # Core
            w216 = refnum<class "AFM_Litho_Plugin.IV.lvclass"> refnum  # Self Reference
            # "lockin Status"
            # "do not delete - used by framework"
            # "Data names and types of shift register data are defined by this bundle."
            # "Initialize the shift-register data, here.\n(data names are defined by what you wire into the bundle function)"
            n76 = Variant To Data(error in=w218, type=w216, Variant=w215) -> (data=w197:refnum<class "AFM_Litho_Plugin.IV.lvclass">, error out=w217:errorcluster)
            n77 = Unbundle By Name(w197) -> ("Lockin Address"=w194:string)
            n78 = Bundle By Name(cluster=w197, "Voltage Channel"=w202) -> (w203:refnum<class "AFM_Litho_Plugin.IV.lvclass">)
            n79 = Variant To Data(type=w195, Variant=w194) -> (data=w196:string)  [unwired: 1 in, 1 out]
            n80 = Bundle By Name(cluster=w203, "Testing?"=w205) -> (w206:refnum<class "AFM_Litho_Plugin.IV.lvclass">)
            n81 = Bundle("Core"=w213, "Self Reference"=w206, "Voltage Channel"=w202, "Lockin Address"=w196, "Plugin Address"=w212, "Server"=w211, "Server Req"=w210, "Server Rep"=w209, "Cycles"=w208, "Status"=Get_State-enum."created", "IV Run"=w207, "IV Status"=w204, "Command History"=w201, "Command Message"=w199, "Start Status"=w198) -> (w219:T12)  [unwired: 1 in]
            n82 = call <vilib>:"Add State(s) to Queue__jki_lib_state_machine.vi"("State(s) in (\"\")"=w221) -> ("States Out"=w220:string)  [unwired: 14 in]
          }
          frame "Data: Cleanup" {
            # "Cleanup any data and references, here.\n(this is called automatically, by the Macro: Exit)"
            n83 = Unbundle By Name(w223) -> ("Core.Current VI Reference"=w226:refnum<vi>)
            n84 = Close Reference(reference=w226, error in (no error)=w225) -> (error out=w224:errorcluster)
            n85 = call <vilib>:"Add State(s) to Queue__jki_lib_state_machine.vi"("State(s) in (\"\")"=w228) -> ("States Out"=w227:string)  [unwired: 14 in]
          }
          frame "---------- UI ----------" {
            # "Do not put any code in this frame.\n(It is a separator no-op. You can make a copy of this frame to create a new UI frame)"
            n86 = call <vilib>:"Add State(s) to Queue__jki_lib_state_machine.vi"("State(s) in (\"\")"=w233) -> ("States Out"=w232:string)  [unwired: 14 in]
          }
          frame "UI: Start Status" {
            # "Do not put any code in this frame.\n(It is a separator no-op. You can make a copy of this frame to create a new UI frame)"
            n87 = Unbundle By Name(w235) -> ("Self Reference"=w242:refnum<class "AFM_Litho_Plugin.IV.lvclass">)
            n88 = Concatenate Strings("Start: " ("string"), w238) -> (w237:string)
            n89 = call "AFM_Litho_Plugin.IV.StartStatus.vi"("error in (no error)"=w240, "StartStatus"=w238, "MeasurementSMO"=w242) -> ("error out"=w241:errorcluster)  [unwired: 7 in, 1 out]
            n90 = Bundle By Name(cluster=w235, "Command Message"=w237) -> (w236:T12)
            n91 = call <vilib>:"Add State(s) to Queue__jki_lib_state_machine.vi"("State(s) in Front (\"\")"="UI: Command History", "State(s) in (\"\")"=w245) -> ("States Out"=w244:string)  [unwired: 13 in]
          }
          frame "UI: Command History" {
            # "12 hours\nHour:Minute:Second"
            # "Make the most recent text black"
            # "Grey out previous commands. Nothing to grey out if first command"
            # "If first command dont put on new line"
            # "Command History"
            # "Put latest command on a new line"
            # "Do not put any code in this frame.\n(It is a separator no-op. You can make a copy of this frame to create a new UI frame)"
            n92 = Unbundle By Name(w262) -> ("Command History"=w246:string, "Command Message"=w249:string)
            n93 = Get Date/Time In Seconds() -> (seconds since 1Jan1904=w254:timestamp)
            n94 = Format Date/Time String(time format string (%c)="%#I:%M:%S", seconds (now)=w254) -> (date/time string=w251:string)  [unwired: 1 in]
            n95 = control-ref of="Incoming Command"() -> (w260:refnum<vi>)
            n96 = Format Into String(format string="%s \\t\\t\\t\\t %s", error in=w248, w249, w251) -> (resulting string=w250:string, error out=w247:errorcluster)  [unwired: 1 in]
            n97 = Empty String/Path?(string/path=w246) -> (empty?=w255:bool)
            n98 = String Length(string=w246) -> (length=w267:i32)
            n99 = case shown="False" w255 {
              tunnel: w267 -> [w277 _]
              tunnel: [w276 w280] -> w265
              tunnel: w247 -> [w275 w280]
              tunnel: w260 -> [w274 w281]
              tunnel: [w273 w281] -> w259
              frame False {
                n100 = property on="Property Node" class="Str"(reference=w274, error in=w275, "Text.Selection Start"=u32 0 ("Text.Selection:Start"), "Text.Selection End"=w277, "Text.FontColor"=u32 8026751 ("Text.Font:Color")) -> (reference out=w273:refnum<vi>, error out=w276:errorcluster)
              }
              frame True {
              }
            }
            n101 = Select(t="", s=w255, f="\r\n") -> (s? t:f=w256:string)
            n102 = Concatenate Strings(w246, w256, w250) -> (w261:string)
            "Incoming Command" <- w261
            n103 = String Length(string=w261) -> (length=w268:i32)
            n104 = Bundle By Name(cluster=w262, "Command History"=w261) -> (w263:T12)
            n105 = property on="Property Node" class="Str"(reference=w259, error in=w265, "Text.Scroll Position"=u32 4294967295, "Text.Selection End"=w268, "Text.Selection Start"=w267, "Text.FontColor"=u32 0 ("Text.Font:Color")) -> (error out=w264:errorcluster)  [unwired: 1 out]
            n106 = call <vilib>:"Add State(s) to Queue__jki_lib_state_machine.vi"("State(s) in (\"\")"=w272) -> ("States Out"=w271:string)  [unwired: 14 in]
          }
          frame "UI: Initialize" {
            # "Initialize the User Interface, here.\n(this is called automatically, by the Macro: Init)"
            n107 = Unbundle By Name(w291) -> ("Lockin Address"=w282:string, "Command History"=w283:string, "Core.Current VI Reference"=w290:refnum<vi>)
            n108 = call <userlib>:"Fit VI window to Largest Dec__ogtk.vi"("error in (no error)"=w292, "border spacing (2 px)"=-3, "VI Ref (calling VI)"=w290) -> ("error out"=w287:errorcluster, "dup VI Ref"=w288:refnum<vi>)  [unwired: 3 in]
            n109 = control-ref of="Incoming Command"() -> (w284:refnum<vi>)
            n110 = property class="VI"(reference=w288, error in=w287, "Front Panel.Resizeable"=FALSE ("Front Panel Window:Resizable")) -> (error out=w286:errorcluster)  [unwired: 1 out]
            n111 = local write "Lock-in Amplifier Address"(w282) -> ()
            n112 = property class="Str"(reference=w284, error in=w286, "Value"=w283) -> (error out=w285:errorcluster)  [unwired: 1 out]
            n113 = call <vilib>:"Add State(s) to Queue__jki_lib_state_machine.vi"("State(s) in (\"\")"=w296) -> ("States Out"=w295:string)  [unwired: 14 in]
          }
          frame "UI: Cursor Set" {
            # "Argument"
            # "Initialize the User Interface, here.\n(this is called automatically, by the Macro: Init)"
            n114 = disable-structure shown="Default" {
              disable-tunnel: w299 -> [w304 w307]
              disable-tunnel: [w304 w306] -> w298
              disable-tunnel: w297 -> [_ w305]
              frame condition #0 {
              }
              frame condition #1 (active) {
                n115 = case shown="\"Idle\", Default" w305 {
                  tunnel: w307 -> [w309 w311]
                  tunnel: [w308 w310] -> w306
                  frame "Idle", Default {
                    n116 = call <vilib>:"Unset Busy.vi"("error in (no error)"=w309) -> ("error out"=w308:errorcluster)  [unwired: 10 in]
                  }
                  frame "Busy" {
                    n117 = call <vilib>:"Set Busy.vi"("error in (no error)"=w311) -> ("error out"=w310:errorcluster)  [unwired: 9 in, 1 out]
                  }
                }
              }
            }
            n118 = call <vilib>:"Add State(s) to Queue__jki_lib_state_machine.vi"("State(s) in (\"\")"=w303) -> ("States Out"=w302:string)  [unwired: 14 in]
          }
          frame "UI: Front Panel State" {
            # "Argument"
            # "Set Front Panel Open or Closed\n(Usage: \"UI: Front Panel State >> Open|Close\")"
            n119 = Unbundle By Name(w315) -> ("Core.Current VI Reference"=w314:refnum<vi>)
            n120 = disable-structure shown="Default" {
              disable-tunnel: w317 -> [w323 w346]
              disable-tunnel: [w322 w346] -> w316
              disable-tunnel: w314 -> [w321 _]
              disable-tunnel: w313 -> [w320 _]
              frame condition #0 (active) {
                n121 = case shown="\"Close\"" w320 {
                  tunnel: w323 -> [w327 w340]
                  tunnel: [w329 w341] -> w322
                  tunnel: w321 -> [w328 w338]
                  frame "Open", Default {
                    n122 = property class="VI"(reference=w328, error in=w327) -> (reference out=w325:refnum<vi>, error out=w326:errorcluster, "FP.State"=w324:T6)
                    n123 = case shown="\"Closed\"" w324 {
                      tunnel: [w332 w335] -> w329
                      tunnel: w326 -> [w331 w335]
                      tunnel: w325 -> [w330 _]
                      frame "Closed" {
                        n124 = invoke class="VI" method="FP.Open"(reference=w330, error in=w331, "Activate"=TRUE, "State"=T6."Standard") -> (error out=w332:errorcluster)  [unwired: 1 in, 4 out]
                      }
                      frame Default {
                      }
                    }
                  }
                  frame "Close" {
                    n125 = property class="VI"(reference=w338, error in=w340) -> (reference out=w337:refnum<vi>, error out=w339:errorcluster, "FP.State"=w336:T6)
                    n126 = case shown="Default" w336 {
                      tunnel: [w342 w345] -> w341
                      tunnel: w339 -> [w342 w344]
                      tunnel: w337 -> [_ w343]
                      frame "Invalid", "Closed" {
                      }
                      frame Default {
                        n127 = invoke class="VI" method="FP.Close"(reference=w343, error in=w344) -> (error out=w345:errorcluster)  [unwired: 1 in, 2 out]
                      }
                    }
                  }
                }
              }
              frame condition #1 {
              }
            }
            n128 = call <vilib>:"Add State(s) to Queue__jki_lib_state_machine.vi"("State(s) in (\"\")"=w319) -> ("States Out"=w318:string)  [unwired: 14 in]
          }
          frame "---------- Macro ----------" {
            # "Do not put any code in this frame.\n(It is a separator no-op. You can make a copy of this frame to create a new Macro frame)"
            n129 = call <vilib>:"Add State(s) to Queue__jki_lib_state_machine.vi"("State(s) in (\"\")"=w351) -> ("States Out"=w350:string)  [unwired: 14 in]
          }
          frame "Macro: IV Progress" {
            # "Do not put any code in this frame.\n(It is a separator no-op. You can make a copy of this frame to create a new Macro frame)"
            n130 = call <vilib>:"Add State(s) to Queue__jki_lib_state_machine.vi"("State(s) in Front (\"\")"="Lockin: Status\nIV: Check Progress", "State(s) in (\"\")"=w357) -> ("States Out"=w356:string)  [unwired: 13 in]
          }
          frame "Macro: Lockin Sweep" {
            # "Do not put any code in this frame.\n(It is a separator no-op. You can make a copy of this frame to create a new Macro frame)"
            n131 = call <vilib>:"Add State(s) to Queue__jki_lib_state_machine.vi"("State(s) in Front (\"\")"="Lockin: Configure Sweep\nLockin: Start Sweep\nLockin: Sweep Started", "State(s) in (\"\")"=w363) -> ("States Out"=w362:string)  [unwired: 13 in]
          }
          frame "Macro: Initialize" {
            w368 = "UI: Start Status >> Connecting to Lockin\nLockin: Open\nServer: Start\nUI: Start Status >> Server Started\nUI: Front Panel State >> Open"  # UI: Start Status >> Connecting to Lockin Lockin: Open Server: Start UI: Start Status >> Server Started UI: Front Panel State >> Open
            w364 = "Process: Sync"
            # "Simplified State Queue\nData: Initialize\nInitialize Core Data\nServer: Create\nEvents: Register\nLockin: Open\nLockin: Get Channels\nServer: Start\nProcess: Sync\nUI: Initialize\nUI: Front Panel State >> Open"
            # "Initialization Macro\n(This is called once, when the VI starts)"
            n132 = control-ref of="This VI"() -> (w366:refnum<vi>)
            n133 = property class="VI"(reference=w366) -> ("Exec.State"=w365:T7)  [unwired: 1 in, 2 out]
            n134 = Equal?(x=w365, y=T7."Run top level") -> (x = y?=w371:bool)
            n135 = Select(t=w364, s=w371, f="") -> ()  [unwired: 1 out]
            n136 = call <vilib>:"Add State(s) to Queue__jki_lib_state_machine.vi"("State(s) in Front (\"\")"="Data: Initialize\nInitialize Core Data\nUI: Initialize\nServer: Create\nUI: Start Status >> Server Created\nEvents: Register\n", "State(s) in (\"\")"=w364, "State(s) at Back (\"\")"=w368) -> ("States Out"=w367:string)  [unwired: 12 in]
            n137 = call <vilib>:"Add State(s) to Queue__jki_lib_state_machine.vi"("State(s) in Front (\"\")"=w367, "State(s) in (\"\")"=w377) -> ("States Out"=w376:string)  [unwired: 13 in]
          }
          frame "Macro: Exit" {
            # "Simplified State Queue\nUI: Front Panel State >> Close\nServer: Stop\nServer: Destroy\nLockin: Close\nData: Cleanup\nEvents: Unregister\nProcess: Sync\nExit"
            # "Exit Macro\n(This is called once, when the VI exits)"
            n138 = Unbundle By Name(w382) -> ("Core.Close Panel on Exit?"=w388:bool)
            n139 = Select(t="UI: Front Panel State >> Close", s=w388, f="") -> (s? t:f=w385:string)
            n140 = call <vilib>:"Add State(s) to Queue__jki_lib_state_machine.vi"("State(s) in Front (\"\")"="Server: Stop\nServer: Destroy\nLockin: Close\nData: Cleanup\nEvents: Unregister", "State(s) in (\"\")"="Process: Sync", "State(s) at Back (\"\")"="Exit") -> ("States Out"=w379:string)  [unwired: 12 in]
            n141 = call <vilib>:"Add State(s) to Queue__jki_lib_state_machine.vi"("State(s) in (\"\")"=w385, "State(s) at Back (\"\")"=w379) -> ("States Out"=w384:string)  [unwired: 13 in]
            n142 = call <vilib>:"Add State(s) to Queue__jki_lib_state_machine.vi"("State(s) in Front (\"\")"=w384, "State(s) in (\"\")"=w391) -> ("States Out"=w390:string)  [unwired: 13 in]
          }
          frame "---------- Process ----------" {
            # "Template Separator\n(You can make a copy of, or modify, this frame)"
            n143 = call <vilib>:"Add State(s) to Queue__jki_lib_state_machine.vi"("State(s) in (\"\")"=w396) -> ("States Out"=w395:string)  [unwired: 14 in]
          }
          frame "Process: Sync" {
            n144 = Unbundle By Name(w404) -> ("Self Reference"=w400:refnum<class "AFM_Litho_Plugin.IV.lvclass">)
            n145 = call <vilib>:"WaitOnProcessSync.vi"("error in (no error)"=w399, "SMO"=w400) -> ("error out"=w398:errorcluster, "Don't run?"=w403:bool)  [unwired: 7 in, 1 out]
            n146 = Select(t="Data: Cleanup\nEvents: Unregister\nExit", s=w403, f="") -> (s? t:f=w397:string)
            n147 = call <vilib>:"Add State(s) to Queue__jki_lib_state_machine.vi"("State(s) in Front (\"\")"=w397, "State(s) in (\"\")"=w407) -> ("States Out"=w406:string)  [unwired: 13 in]
          }
          frame "---------- Events ----------" {
            # "Template Separator\n(You can make a copy of, or modify, this frame)"
            n148 = call <vilib>:"Add State(s) to Queue__jki_lib_state_machine.vi"("State(s) in (\"\")"=w412) -> ("States Out"=w411:string)  [unwired: 14 in]
          }
          frame "Events: Register" {
            # "Expand to add\nmore events"
            n149 = Unbundle By Name(w419) -> ("Self Reference"=w415:refnum<class "AFM_Litho_Plugin.IV.lvclass">)
            n150 = Unbundle By Name(w419) -> ("Server"=w416:refnum<class "RemoteControl.lvclass">)
            n151 = call <userlib>:"RemoteControl.GetPublicEvents.vi"("RemoteControl"=w416) -> ("error out"=w418:errorcluster, "RC Public Events"=w417:T14)  [unwired: 8 in, 1 out]
            n152 = call "AFM_Litho_Plugin.IV.GetPrivateEvents.vi"("MeasurementSMO"=w415) -> ("error out"=w413:errorcluster, "Private Events"=w414:T15)  [unwired: 8 in, 1 out]
            n153 = call <vilib>:"GetProtectedEvents.vi"("SMO"=w415) -> ("error out"=w420:errorcluster, "SMO Protected Events"=w424:T16)  [unwired: 8 in, 1 out]
            n154 = register-events(w424, w417, w414) -> (reference out=w425:refnum<event-registration>, error out=w421:errorcluster)  [unwired: 2 in]
            n155 = Merge Errors(w423, w421, w420, w418, w413) -> (w422:errorcluster)
            n156 = call <vilib>:"Add State(s) to Queue__jki_lib_state_machine.vi"("State(s) in (\"\")"=w427) -> ("States Out"=w426:string)  [unwired: 14 in]
          }
          frame "Events: Unregister" {
            n157 = Unregister For Events(event registration refnum=w430, error in=w429) -> (error out=w428:errorcluster)
            n158 = call <vilib>:"Clear Errors.vi"("error in (no error)"=w428) -> ()  [unwired: 5 in, 2 out]
            n159 = call <vilib>:"Add State(s) to Queue__jki_lib_state_machine.vi"("State(s) in (\"\")"=w433) -> ("States Out"=w432:string)  [unwired: 14 in]
          }
          frame "---------- Lockin ----------" {
            n160 = Unbundle By Name(w435) -> ("Self Reference"=w434:refnum<class "AFM_Litho_Plugin.IV.lvclass">)
            n161 = Bundle By Name(cluster=w435, "Self Reference"=w434) -> (w436:T12)
            n162 = call <vilib>:"Add State(s) to Queue__jki_lib_state_machine.vi"("State(s) in (\"\")"=w440) -> ("States Out"=w439:string)  [unwired: 14 in]
          }
          frame "Lockin: Open" {
            # "#todo\nMake a way to attempt to connect after notifying user if lockin is not connected\nReturn Errors to external commands if lockin is not connected"
            n163 = Unbundle By Name(w451) -> ("Self Reference"=w450:refnum<class "AFM_Litho_Plugin.IV.lvclass">, "Lockin Address"=w446:string)
            n164 = call "Open Lockin.vi"("error in (no error)"=w449, "Lockin Address"=w446, "MeasurementSMO in"=w450) -> ("error out"=w448:errorcluster, "Connected?"=w445:bool, "MeasurementSMO out"=w447:refnum<class "AFM_Litho_Plugin.IV.lvclass">)  [unwired: 5 in, 1 out]
            "Lock-in Connection" <- w445
            n165 = Select(t="Lockin: Get Channels", s=w445, f="UI: Start Status >> Lockin Connection Failed") -> (s? t:f=w443:string)
            n166 = Bundle By Name(cluster=w451, "Self Reference"=w447) -> (w452:T12)
            n167 = call <vilib>:"Add State(s) to Queue__jki_lib_state_machine.vi"("State(s) in Front (\"\")"=w443, "State(s) in (\"\")"=w442) -> ("States Out"=w454:string)  [unwired: 13 in]
          }
          frame "Lockin: Get Sweep Data" {
            n168 = Unbundle By Name(w463) -> ("Self Reference"=w462:refnum<class "AFM_Litho_Plugin.IV.lvclass">)
            n169 = call "Get Lockin Sweep Data.vi"("error in (no error)"=w461, "MeasurementSMO in"=w462) -> ("error out"=w456:errorcluster, "Sweep_AI"=w457:waveform(dbl)[], "Sweep_AO"=w458:waveform(dbl)[], "MeasurementSMO out"=w460:refnum<class "AFM_Litho_Plugin.IV.lvclass">)  [unwired: 6 in]
            n170 = call "SaveLockinSweepData.vi"("error in (no error)"=w456, "Sweep_AI"=w457, "Sweep_AO"=w458, "AFM_Litho_Plugin.IV in"=w460) -> ("error out"=w455:errorcluster, "AFM_Litho_Plugin.IV out"=w459:refnum<class "AFM_Litho_Plugin.IV.lvclass">)  [unwired: 6 in]
            n171 = Bundle By Name(cluster=w463, "Self Reference"=w459) -> (w464:T12)
            n172 = call <vilib>:"Add State(s) to Queue__jki_lib_state_machine.vi"("State(s) in (\"\")"=w467) -> ("States Out"=w466:string)  [unwired: 14 in]
          }
          frame "Lockin: Get Channels" {
            # "Populate a list of possible outputs to sweep.\nInputs are configured in Lockin program."
            n173 = Unbundle By Name(w475) -> ("Self Reference"=w474:refnum<class "AFM_Litho_Plugin.IV.lvclass">)
            n174 = call "Get Lockin Channels.vi"("error in (no error)"=w472, "MeasurementSMO in"=w474) -> ("error out"=w469:errorcluster, "size(s)"=w471:i32, "MeasurementSMO out"=w473:refnum<class "AFM_Litho_Plugin.IV.lvclass">)  [unwired: 6 in, 1 out]
            n175 = for {
              N: w471 -> [_]
              tunnel: [w482] -> w470 mode=indexing
              i -> [w484]
              n176 = Increment(x=w484) -> (x+1=w481:i32)
              n177 = Number To Decimal String(number=w481) -> (decimal integer string=w480:string)  [unwired: 1 in]
              n178 = Concatenate Strings("ao" ("string"), w480) -> (w482:string)
            }
            n179 = property on="Output Channel" class="Ring (strict)"(error in=w469, "Strings []"=w470) -> (error out=w468:errorcluster)  [unwired: 1 in, 1 out]
            n180 = Bundle By Name(cluster=w475, "Self Reference"=w473) -> (w476:T12)
            n181 = call <vilib>:"Add State(s) to Queue__jki_lib_state_machine.vi"("State(s) in (\"\")"=w479) -> ("States Out"=w478:string)  [unwired: 14 in]
          }
          frame "Lockin: Set IV Mode" {
            # "This is no longer called. From a previous version of the lockin program."
            n182 = Unbundle By Name(w487) -> ("Self Reference"=w485:refnum<class "AFM_Litho_Plugin.IV.lvclass">)
            n183 = Match True/False String(2:"FALSE" ("false string"), 3:"TRUE" ("true string"), 4:w492) -> (0:w489:bool)  [unwired: 1 out]
            n184 = call "Set Lockin IV Mode.vi"("error in (no error)"=w493, "IV Mode?"=w489, "MeasurementSMO in"=w485) -> ("error out"=w494:errorcluster, "MeasurementSMO out"=w486:refnum<class "AFM_Litho_Plugin.IV.lvclass">)  [unwired: 7 in]
            n185 = Bundle By Name(cluster=w487, "Self Reference"=w486) -> (w488:T12)
            n186 = call <vilib>:"Add State(s) to Queue__jki_lib_state_machine.vi"("State(s) in (\"\")"=w497) -> ("States Out"=w496:string)  [unwired: 14 in]
          }
          frame "Lockin: Configure Sweep" {
            n187 = Unbundle By Name(w498) -> ("Self Reference"=w503:refnum<class "AFM_Litho_Plugin.IV.lvclass">, "IV Run"=w501:T3)
            n188 = call "Configure Lockin.vi"("error in (no error)"=w500, "IV Run"=w501, "MeasurementSMO in"=w503) -> ("error out"=w499:errorcluster, "MeasurementSMO out"=w502:refnum<class "AFM_Litho_Plugin.IV.lvclass">)  [unwired: 7 in]
            n189 = Bundle By Name(cluster=w498, "Self Reference"=w502) -> (w504:T12)
            n190 = call <vilib>:"Add State(s) to Queue__jki_lib_state_machine.vi"("State(s) in (\"\")"=w507) -> ("States Out"=w506:string)  [unwired: 14 in]
          }
          frame "Lockin: Start Sweep" {
            n191 = Unbundle By Name(w512) -> ("Self Reference"=w511:refnum<class "AFM_Litho_Plugin.IV.lvclass">)
            n192 = call "Start Lockin Sweep.vi"("error in (no error)"=w509, "MeasurementSMO in"=w511) -> ("error out"=w508:errorcluster, "MeasurementSMO out"=w510:refnum<class "AFM_Litho_Plugin.IV.lvclass">)  [unwired: 8 in]
            n193 = Bundle By Name(cluster=w512, "Self Reference"=w510) -> (w513:T12)
            n194 = call <vilib>:"Add State(s) to Queue__jki_lib_state_machine.vi"("State(s) in (\"\")"=w516) -> ("States Out"=w515:string)  [unwired: 14 in]
          }
          frame "Lockin: Sweep Started" {
            n195 = Unbundle By Name(w522) -> ("Self Reference"=w521:refnum<class "AFM_Litho_Plugin.IV.lvclass">)
            n196 = call "Wait Lockin Start.vi"("error in (no error)"=w519, "MeasurementSMO in"=w521) -> ("error out"=w518:errorcluster, "MeasurementSMO out"=w520:refnum<class "AFM_Litho_Plugin.IV.lvclass">)  [unwired: 8 in]
            n197 = Bundle By Name(cluster=w522, "Self Reference"=w520, "IV Status"="RUNNING") -> (w523:T12)
            n198 = call <vilib>:"Add State(s) to Queue__jki_lib_state_machine.vi"("State(s) in (\"\")"=w526) -> ("States Out"=w525:string)  [unwired: 14 in]
          }
          frame "Lockin: Stop Sweep" {
            n199 = Unbundle By Name(w532) -> ("Self Reference"=w534:refnum<class "AFM_Litho_Plugin.IV.lvclass">)
            n200 = call "Stop Lockin Sweep.vi"("error in (no error)"=w528, "MeasurementSMO in"=w534) -> ("error out"=w529:errorcluster, "MeasurementSMO out"=w531:refnum<class "AFM_Litho_Plugin.IV.lvclass">)  [unwired: 8 in]
            n201 = Bundle By Name(cluster=w532, "Self Reference"=w531, "Cycles"=0.0 ("IV Run.Cycles"), "IV Status"="ABORTED") -> (w533:T12)
            n202 = call <vilib>:"Add State(s) to Queue__jki_lib_state_machine.vi"("State(s) in (\"\")"=w537) -> ("States Out"=w536:string)  [unwired: 14 in]
          }
          frame "Lockin: Status" {
            n203 = Unbundle By Name(w543) -> ("Self Reference"=w540:refnum<class "AFM_Litho_Plugin.IV.lvclass">)
            n204 = call "Get Lockin Status.vi"("error in (no error)"=w542, "MeasurementSMO in"=w540) -> ("error out"=w541:errorcluster, "Status"=w538:T5, "MeasurementSMO out"=w539:refnum<class "AFM_Litho_Plugin.IV.lvclass">)  [unwired: 7 in]
            n205 = Bundle By Name(cluster=w543, "Self Reference"=w539, "Status"=w538) -> (w544:T12)
            n206 = call <vilib>:"Add State(s) to Queue__jki_lib_state_machine.vi"("State(s) in (\"\")"=w547) -> ("States Out"=w546:string)  [unwired: 14 in]
          }
          frame "Lockin: Close" {
            n207 = Unbundle By Name(w552) -> ("Self Reference"=w549:refnum<class "AFM_Litho_Plugin.IV.lvclass">)
            n208 = call "Close Lockin.vi"("error in (no error)"=w551, "MeasurementSMO in"=w549) -> ("error out"=w550:errorcluster, "MeasurementSMO out"=w548:refnum<class "AFM_Litho_Plugin.IV.lvclass">)  [unwired: 8 in]
            n209 = Bundle By Name(cluster=w552, "Self Reference"=w548) -> (w553:T12)
            n210 = call <vilib>:"Add State(s) to Queue__jki_lib_state_machine.vi"("State(s) in (\"\")"=w556) -> ("States Out"=w555:string)  [unwired: 14 in]
          }
          frame "---------- Server ----------" {
            # "The server in this case is the plugin's Remote Control Server.\nThis is the way that the lithography program interfaces with the Plugin"
            n211 = Unbundle By Name(w558) -> ("Server"=w557:refnum<class "RemoteControl.lvclass">)
            n212 = Bundle By Name(cluster=w558, "Server"=w557) -> (w559:T12)
            n213 = call <vilib>:"Add State(s) to Queue__jki_lib_state_machine.vi"("State(s) in (\"\")"=w563) -> ("States Out"=w562:string)  [unwired: 14 in]
          }
          frame "Server: Reply" {
            # "Blank out request as we have fulfilled what has been requested"
            n214 = Unbundle By Name(w570) -> ("Server"=w569:refnum<class "RemoteControl.lvclass">, "Server Rep"=w567:T11)
            n215 = call <userlib>:"RemoteControl.SendMessageToProcess.vi"("error in (no error)"=w565, "SendMessageToProcess"=w567, "RemoteControl"=w569) -> ("error out"=w566:errorcluster, "RemoteControl out"=w568:refnum<class "RemoteControl.lvclass">)  [unwired: 7 in]
            n216 = Bundle By Name(cluster=w570, "Server"=w568, "Server Req"=T8 {"Command"="", "Data"=variant, "ID"=""}) -> (w571:T12)
            n217 = call <vilib>:"Add State(s) to Queue__jki_lib_state_machine.vi"("State(s) in (\"\")"=w574) -> ("States Out"=w573:string)  [unwired: 14 in]
          }
          frame "Server: Create" {
            n218 = Unbundle By Name(w592) -> ("Self Reference"=w576:refnum<class "AFM_Litho_Plugin.IV.lvclass">)
            n219 = Unbundle By Name(w576) -> ("Plugin Port"=w575:u16)
            "IV Plug-in Address" <- w575
            n220 = call <userlib>:"RC Enum to RC Object.vi"("error in (no error)"=w577, "RC Type"=RC_Com_Type--enum."ZMQ") -> ("error out"=w585:errorcluster, "RemoteControl out"=w586:refnum<class "RemoteControl.lvclass">)  [unwired: 8 in]
            n221 = call-dynamic "Write address.vi"("error in (no error)"=w585, "address"="", "RemoteControl in"=w586) -> ("error out"=w589:errorcluster, "RemoteControl out"=w590:refnum<class "RemoteControl.lvclass">)  [unwired: 7 in]
            n222 = call-dynamic "Write Port.vi"("error in (no error)"=w589, "Port"=w575, "RemoteControl in"=w590) -> ("error out"=w587:errorcluster, "RemoteControl out"=w588:refnum<class "RemoteControl.lvclass">)  [unwired: 7 in]
            n223 = call-dynamic "Write Commands.vi"("error in (no error)"=w587, "Commands"=string[] ["ACK", "HELP", "IV_RUN", "IV_STATUS", "IV_ABORT"], "RemoteControl in"=w588) -> ("error out"=w579:errorcluster, "RemoteControl out"=w581:refnum<class "RemoteControl.lvclass">)  [unwired: 7 in]
            n224 = call-dynamic "Create Server SMO.vi"("error in (no error)"=w579, "RemoteControl in"=w581) -> ("error out"=w578:errorcluster, "RemoteControl out"=w580:refnum<class "RemoteControl.lvclass">)  [unwired: 8 in]
            n225 = Bundle By Name(cluster=w592, "Server"=w580) -> (w591:T12)
            n226 = call <vilib>:"Add State(s) to Queue__jki_lib_state_machine.vi"("State(s) in (\"\")"=w595) -> ("States Out"=w594:string)  [unwired: 14 in]
          }
          frame "Server: Start" {
            n227 = Unbundle By Name(w597) -> ("Server"=w601:refnum<class "RemoteControl.lvclass">)
            n228 = call <vilib>:"Start.vi"("error in (no error)"=w599, "SMO"=w601) -> ("error out"=w600:errorcluster, "SMO out"=w596:refnum<class "RemoteControl.lvclass">)  [unwired: 8 in]
            n229 = Bundle By Name(cluster=w597, "Server"=w596) -> (w598:T12)
            n230 = call <vilib>:"Add State(s) to Queue__jki_lib_state_machine.vi"("State(s) in (\"\")"=w604) -> ("States Out"=w603:string)  [unwired: 14 in]
          }
          frame "Server: Stop" {
            # "The server in this case is the plugin's Remote Control Server.\nThis is the way that the lithography program interfaces with the Plugin"
            n231 = Unbundle By Name(w609) -> ("Server"=w608:refnum<class "RemoteControl.lvclass">)
            n232 = call <vilib>:"Stop.vi"("error in (no error)"=w605, "SMO"=w608) -> ("error out"=w606:errorcluster, "SMO out"=w607:refnum<class "RemoteControl.lvclass">)  [unwired: 8 in]
            n233 = Bundle By Name(cluster=w609, "Server"=w607) -> (w610:T12)
            n234 = call <vilib>:"Add State(s) to Queue__jki_lib_state_machine.vi"("State(s) in (\"\")"=w613) -> ("States Out"=w612:string)  [unwired: 14 in]
          }
          frame "Server: Destroy" {
            # "The server in this case is the plugin's Remote Control Server.\nThis is the way that the lithography program interfaces with the Plugin"
            n235 = Unbundle By Name(w618) -> ("Server"=w616:refnum<class "RemoteControl.lvclass">)
            n236 = call <vilib>:"Destroy.vi"("error in (no error)"=w614, "SMO"=w616) -> ("error out"=w615:errorcluster)  [unwired: 9 in]
            n237 = Bundle By Name(cluster=w618, "Server"=refnum<class "RemoteControl.lvclass"> refnum) -> (w619:T12)
            n238 = call <vilib>:"Add State(s) to Queue__jki_lib_state_machine.vi"("State(s) in (\"\")"=w622) -> ("States Out"=w621:string)  [unwired: 14 in]
          }
          frame "---------- Remote ----------" {
            n239 = Unbundle By Name(w623) -> ("Server Req.Command"=w627:string)
            n240 = call <vilib>:"Build State String with Arguments__JKI_lib_State_Machine.vi"("Arguments (\"\")"=w627, "State"="Remote: Format") -> ("State with Arguments"=w626:string)  [unwired: 4 in]
            n241 = call <vilib>:"Add State(s) to Queue__jki_lib_state_machine.vi"("State(s) in (\"\")"=w626, "State(s) at Back (\"\")"="Server: Reply" ("State(s) at Back (\"\")")) -> ("States Out"=w624:string)  [unwired: 13 in]
            n242 = call <vilib>:"Add State(s) to Queue__jki_lib_state_machine.vi"("State(s) in Front (\"\")"=w624, "State(s) in (\"\")"=w632) -> ("States Out"=w631:string)  [unwired: 13 in]
          }
          frame "Remote: Format" {
            # "Formats a reply for an incoming command."
            n243 = Unbundle By Name(w636) -> ("Server Req.Command"=w635:string, "Server Req.ID"=w634:string)
            n244 = case shown="\"IV_STATUS\"" w638 {
              tunnel: w636 -> [_ _ _ _ _ w654]
              tunnel: [variant "RUNNING" w646 "ABORTED" string[] ["IV_RUN", "IV_STATUS", "IV_ABORT", "ACK", "HELP"] w652] -> w633
              frame Default {
              }
              frame "IV_RUN" {
              }
              frame "ACK" {
                n245 = Get Date/Time In Seconds() -> (seconds since 1Jan1904=w647:timestamp)
                n246 = Format Date/Time String(time format string (%c)="%H:%M:%S", seconds (now)=w647) -> (date/time string=w648:string)  [unwired: 1 in]
                n247 = Concatenate Strings("OK " ("data"), w648) -> (w646:string)
              }
              frame "IV_ABORT" {
              }
              frame "HELP" {
              }
              frame "IV_STATUS" {
                n248 = Unbundle By Name(w654) -> ("IV Status"=w653:string)
                n249 = To Upper Case(1:w653) -> (0:w652:string)
              }
            }
            n250 = Bundle By Name(cluster=w636, "Server Rep.Message.Command"=w635, "Server Rep.Message.ID"=w634, "Server Rep.Message.Data"=w633) -> (w637:T12)
            n251 = call <vilib>:"Add State(s) to Queue__jki_lib_state_machine.vi"("State(s) in (\"\")"=w642) -> ("States Out"=w641:string)  [unwired: 14 in]
          }
          frame "Remote: ACK" {
            # "Simplified State Queue\nRemote: Format >> ACK\nServer: Reply"
            n252 = Unbundle By Name(w655) -> ("Server Req.Command"=w659:string)
            n253 = call <vilib>:"Build State String with Arguments__JKI_lib_State_Machine.vi"("Arguments (\"\")"=w659, "State"="Remote: Format") -> ("State with Arguments"=w658:string)  [unwired: 4 in]
            n254 = call <vilib>:"Add State(s) to Queue__jki_lib_state_machine.vi"("State(s) in (\"\")"=w658, "State(s) at Back (\"\")"="Server: Reply" ("State(s) at Back (\"\")")) -> ("States Out"=w656:string)  [unwired: 13 in]
            n255 = call <vilib>:"Add State(s) to Queue__jki_lib_state_machine.vi"("State(s) in Front (\"\")"=w656, "State(s) in (\"\")"=w664) -> ("States Out"=w663:string)  [unwired: 13 in]
          }
          frame "Remote: HELP" {
            # "Simplified State Queue\nRemote: Format >> HELP\nServer: Reply"
            n256 = Unbundle By Name(w666) -> ("Server Req.Command"=w669:string)
            n257 = call <vilib>:"Build State String with Arguments__JKI_lib_State_Machine.vi"("Arguments (\"\")"=w669, "State"="Remote: Format") -> ("State with Arguments"=w668:string)  [unwired: 4 in]
            n258 = call <vilib>:"Add State(s) to Queue__jki_lib_state_machine.vi"("State(s) in (\"\")"=w668, "State(s) at Back (\"\")"="Server: Reply" ("State(s) at Back (\"\")")) -> ("States Out"=w665:string)  [unwired: 13 in]
            n259 = call <vilib>:"Add State(s) to Queue__jki_lib_state_machine.vi"("State(s) in Front (\"\")"=w665, "State(s) in (\"\")"=w674) -> ("States Out"=w673:string)  [unwired: 13 in]
          }
          frame "Remote: IV_ABORT" {
            # "Simplified State Queue\nLockin: Stop Sweep //if sweep isnt finished\n//Lockin: Set IV Mode >> False\nRemote: Format >> IV_ABORT\nServer: Reply"
            # "Prevent timeout from calling next cycle"
            # "If it is finished we shouldnt need to send abort command"
            n260 = Unbundle By Name(w685) -> ("IV Status"=w682:string, "Server Req.Command"=w675:string)
            n261 = Bundle By Name(cluster=w685, "Cycles"=0.0) -> (w686:T12)
            n262 = To Upper Case(1:w682) -> (0:w677:string)
            n263 = Not Equal?(x="FINISHED", y=w677) -> (x != y?=w681:bool)
            n264 = call <vilib>:"Build State String with Arguments__JKI_lib_State_Machine.vi"("Arguments (\"\")"=w675, "State"="Remote: Format") -> ("State with Arguments"=w688:string)  [unwired: 4 in]
            n265 = Select(t="Lockin: Stop Sweep\n//Lockin: Set IV Mode >> FALSE", s=w681, f="") -> (s? t:f=w678:string)
            n266 = call <vilib>:"Add State(s) to Queue__jki_lib_state_machine.vi"("State(s) in Front (\"\")"=w678, "State(s) in (\"\")"=w688, "State(s) at Back (\"\")"="Server: Reply" ("State(s) at Back (\"\")")) -> ("States Out"=w687:string)  [unwired: 12 in]
            n267 = call <vilib>:"Add State(s) to Queue__jki_lib_state_machine.vi"("State(s) in Front (\"\")"=w687, "State(s) in (\"\")"=w693) -> ("States Out"=w692:string)  [unwired: 13 in]
          }
          frame "Remote: IV_RUN" {
            # "Simplified State Queue\n//Lockin: Set IV Mode >> TRUE\nMacro: Lockin Sweep\nRemote: Format >> IV_RUN\nServer: Reply"
            n268 = Unbundle By Name(w695) -> ("Server Req.Command"=w706:string, "IV Run"=w698:T3, "Server"=w697:refnum<class "RemoteControl.lvclass">, "Server Req.Data"=w694:variant)
            n269 = Variant To Data(error in=w709, type="", Variant=w694) -> (data=w707:string, error out=w704:errorcluster)
            n270 = call "Variant to Data.vim"("Data Type"=w698, "error in (no error)"=w704, "Data in"=w707, "RemoteControl in"=w697) -> ("error out"=w703:errorcluster, "Data out"=w705:T3)  [unwired: 5 in, 1 out]
            n271 = Unbundle By Name(w705) -> ("Cycles"=w696:dbl, "Rate"=→"Rate":dbl, "End"=→"End":dbl, "Start"=→"Start":dbl, "Pattern"=→"Pattern":T1)
            "Cycles" <- w696
            n272 = Bundle By Name(cluster=w695, "IV Run"=w705, "Cycles"=w696) -> (w710:T12)
            n273 = call <vilib>:"Build State String with Arguments__JKI_lib_State_Machine.vi"("Arguments (\"\")"=w706, "State"="Remote: Format") -> ("State with Arguments"=w713:string)  [unwired: 4 in]
            n274 = call <vilib>:"Add State(s) to Queue__jki_lib_state_machine.vi"("State(s) in Front (\"\")"="//Lockin: Set IV Mode >> TRUE\nMacro: Lockin Sweep", "State(s) in (\"\")"=w713, "State(s) at Back (\"\")"="Server: Reply" ("State(s) at Back (\"\")")) -> ("States Out"=w712:string)  [unwired: 12 in]
            n275 = call <vilib>:"Add State(s) to Queue__jki_lib_state_machine.vi"("State(s) in Front (\"\")"=w712, "State(s) in (\"\")"=w718) -> ("States Out"=w717:string)  [unwired: 13 in]
          }
          frame "Remote: IV_STATUS" {
            # "Simplified State Queue\nMacro: IV Progress\nRemote: Format >> IV_STATUS\nServer: Reply"
            n276 = Unbundle By Name(w723) -> ("Server Req.Command"=w721:string)
            n277 = call <vilib>:"Build State String with Arguments__JKI_lib_State_Machine.vi"("Arguments (\"\")"=w721, "State"="Remote: Format") -> ("State with Arguments"=w722:string)  [unwired: 4 in]
            n278 = call <vilib>:"Add State(s) to Queue__jki_lib_state_machine.vi"("State(s) in Front (\"\")"="Macro: IV Progress", "State(s) in (\"\")"=w722, "State(s) at Back (\"\")"="Server: Reply" ("State(s) at Back (\"\")")) -> ("States Out"=w719:string)  [unwired: 12 in]
            n279 = call <vilib>:"Add State(s) to Queue__jki_lib_state_machine.vi"("State(s) in Front (\"\")"=w719, "State(s) in (\"\")"=w729) -> ("States Out"=w728:string)  [unwired: 13 in]
          }
          frame "---------- IV ----------" {
            n280 = call <vilib>:"Add State(s) to Queue__jki_lib_state_machine.vi"("State(s) in (\"\")"=w734) -> ("States Out"=w733:string)  [unwired: 14 in]
          }
          frame "IV: Finished Cycle" {
            # "Simplified State Queue\nIf finished:\n//Lockin: Set IV Mode >> FALSE\n[state queue]\nLockin: Get Sweep Data\n\nIf not finished:\nMacro: Lockin Sweep"
            # "Get Sweep Data"
            # "No more cycles to do"
            # "Subtract off the finished cycle."
            # "There are more cycles to do..."
            n281 = Unbundle By Name(w746) -> ("Cycles"=w748:dbl, "IV Status"=w736:string)
            n282 = Decrement(x=w748) -> (x-1=w740:dbl)
            n283 = Less Or Equal To 0?(x=w740) -> (x <= 0?=w735:bool)
            n284 = Select(t="Finished", s=w735, f=w736) -> (s? t:f=w741:string)
            n285 = Bundle By Name(cluster=w746, "Cycles"=w740, "IV Status"=w741) -> (w747:T12)
            n286 = Select(t="//Lockin: Set IV Mode >> FALSE", s=w735, f="Macro: Lockin Sweep") -> (s? t:f=w744:string)
            n287 = Select(t="Lockin: Get Sweep Data", s=w735, f="") -> (s? t:f=w737:string)
            n288 = call <vilib>:"Add State(s) to Queue__jki_lib_state_machine.vi"("State(s) in Front (\"\")"=w744, "State(s) in (\"\")"=w752, "State(s) at Back (\"\")"=w737) -> ("States Out"=w751:string)  [unwired: 12 in]
          }
          frame "IV: Check Progress" {
            # "IDLE means that there hasn't been a curve started yet. Don't bother checking (its not designed to check if the cycle is finished yet if it is in an idle state."
            # "If it is already Finished, you should not call IV: Finished Cycle because thats just a status call from the Remote Process"
            # "Simplified State Queue\nIV: Finished Cycle"
            # "Calling abort causes issues with this state."
            n289 = Unbundle By Name(w765) -> ("Status"=w768:T5, "IV Status"=w762:string)
            n290 = To Upper Case(1:w762) -> (0:w760:string)
            n291 = Not Equal?(x=Get_State-enum."sweeping" ("Status"), y=w768) -> (x != y?=w758:bool)
            n292 = Not Equal?(x=w760, y="ABORTED") -> (x != y?=w757:bool)
            n293 = Not Equal?(x=w760, y="IDLE") -> (x != y?=w756:bool)
            n294 = Not Equal?(x=w760, y="FINISHED") -> (x != y?=w755:bool)
            n295 = Compound Arithmetic op=AND(w758, w757, w756, w755) -> (w754:bool)
            n296 = Select(t="IV: Finished Cycle", s=w754, f="") -> (s? t:f=w763:string)
            n297 = call <vilib>:"Add State(s) to Queue__jki_lib_state_machine.vi"("State(s) in Front (\"\")"=w763, "State(s) in (\"\")"=w772) -> ("States Out"=w771:string)  [unwired: 13 in]
          }
        }
      }
    }
    frame Error {
    }
  }
  n298 = call-parent "Process.vi"("error in (no error)"=w7, "SMO.UI"=w6) -> ("error out"=w4:errorcluster, "SMO.UI out"=→"MeasurementSMO out":refnum<class "AFM_Litho_Plugin.IV.lvclass">)  [unwired: 8 in]
  n299 = Merge Errors(w4, w3) -> (→"error out":errorcluster)
